vi "HMI_Prototype.vi"() -> ()   [LabVIEW 2014]
uses:
  machineState.ctl
  controls.ctl
  <vilib>/DAQmx/write.llb/DAQmx Write (Digital Bool 1Line 1Point).vi
  <vilib>/DAQmx/read.llb/DAQmx Read (Analog DBL 1Chan 1Samp).vi
  <vilib>/DAQmx/miscellaneous.llb/DAQmx Fill In Error Info.vi
panel:
  out "lab":dbl
  out "solution":dbl
  out "Issue Resolved:":bool
  out "Budget:":dbl=800.0 format="$%#_g.00"
  out "Time Remaining:":timestamp=timestamp(1800 s since 1904-01-01) format="%<%M:%S>T"
  in  "Terminal:":T1(ring)
  in  "Component:":T2(ring)
  in  "Tighten Terminal":bool
  in  "Replace Component":bool
  in  "Segment:":T3(ring)
  in  "Aquire Voltage":bool
  out "Voltage:":dbl
  out "Lab:":string
  in  "Close Lab":bool
  in  "Reset Lab":bool
  out "V+ Solenoid":bool
  out "B+ Solenoid":bool
  out "A- Solenoid":bool
  out "A+ Solenoid":bool
  out "Manual":bool
  out "Auto":bool=TRUE
  out "Stop Button":bool
  out "Start Button":bool
  in  "Tab Control":T4(tab)
  in  "WebBrowser":refnum<k7>(container)
  out "s1":picture
  out "s2":picture
  out "s3":picture
  out "s4":picture
  in  "V+":bool
  in  "B+":bool
  in  "A-":bool
  in  "A+":bool
  in  "START":bool
  in  "AUTO/MAN":bool
  in  "STOP":bool
  # "A+"
  # "A-"
  # "B+"
  # "V+"
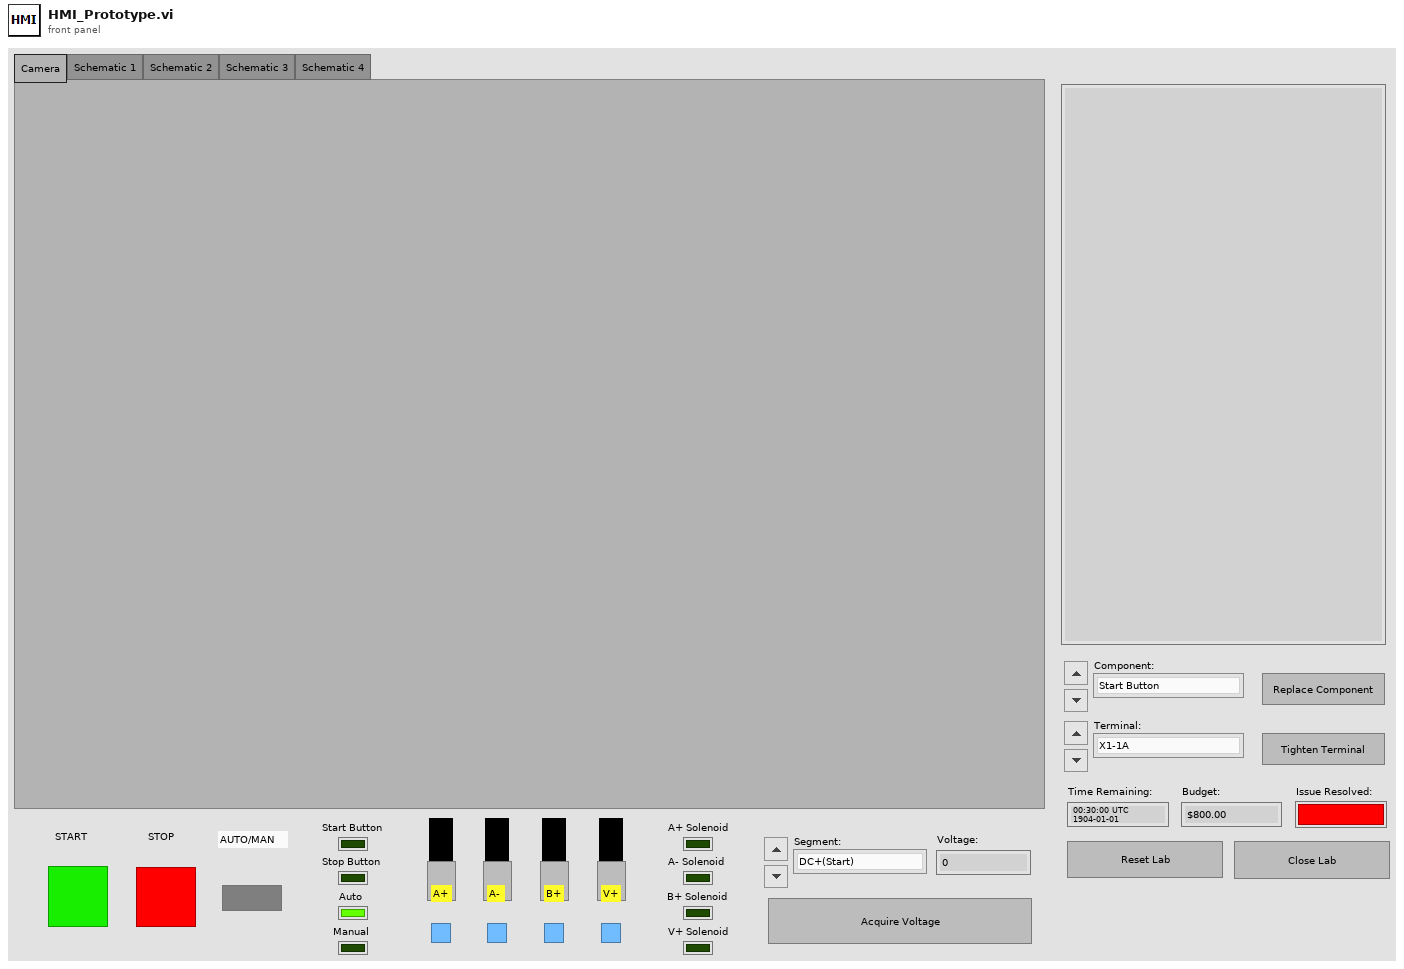
[diagram p1: front panel]
types:
  T1 = enum16{"X1-1A", "X1-2A", "X1-3A", "X1-4A", "X1-5A", "X1-6A", "X1-7A", "X1-8A", "X1-9A", "X1-10A", "X1-11A", "X1-12A", "X1-1B", "X1-2B", "X1-3B", "X1-4B", "X1-5B", "X1-6B", "X1-7B", "X1-8B", "X1-9B", "X1-10B", "X1-11B", "X1-12B", "X1-1C", "X1-2C", "X1-3C", "X1-4C", "X1-5C", "X1-6C", "X1-7C", "X1-8C", "X1-9C", "X1-10C", "X1-11C", "X1-12C", "X1-1D", "X1-2D", "X1-3D", "X1-4D", "X1-5D", "X1-6D", "X1-7D", "X1-8D", "X1-9D", "X1-10D", "X1-11D", "X1-12D", "PLC-VDC(O/0)", "PLC-O/0", "PLC-VDC(O/1)", "PLC-O/1", "PLC-VDC(O/2)", "PLC-O/2", "PLC-VDC(O/3)", "PLC-O/3", "PLC-DC_COM1", "PLC-I/0", "PLC-I/1", "PLC-I/2", "PLC-I/3", "PLC-DC_COM2", "PLC-I/4", "PLC-I/5", "PLC-I/6", "PLC-I/7", "Start Button Terminals", "Stop Button Terminals", "Auto/Man Terminals", "DM1(a0) Terminals", "DM2(a1) Terminals", "DM3(b0) Terminals", "DM4(b1) Terminals", "DM5(v) Terminals", "EL1(A+) Terminals", "EL2(A-) Terminals", "EL3(B+) Terminals", "EL4(V+) Terminals"}
  T2 = enum16{"Start Button", "Stop Button", "Auto/Man Switch", "DM1(a0)", "DM2(a1)", "DM3(b0)", "DM4(b1)", "DM5(v)", "EL1(A+)", "EL2(A-)", "EL3(B+)", "EL4(V+)", "PLC"}
  T3 = enum16{"DC+(Start)", "PB(Start)", "I/0(Start)", "DC+(Stop)", "PB(Stop)", "I/1(Stop)", "DC+(Auto/Man)", "I/2(Auto/Man)", "DC+(a0)", "I/3(a0)", "DC+(a1)", "I/4(a1)", "DC+(b0)", "I/5(b0)", "DC+(b1)", "I/6(b1)", "DC+(v)", "I/7(v)", "DC+(O/0)(VAC/VDC)", "O/0(EL1A+)", "EL1A+(A1)", "EL1A+(A2)", "DC+(O/1)(VAC/VDC)", "O/1(EL2A-)", "EL2A-(A1)", "EL2A-(A2)", "O/2(EL3B+)(A1)", "EL3B+(A2)", "O/3(EL4V+)(A1)", "EL4V+(A2)", "DC-(DC_COM)", "DC-(0V)"}
  T4 = enum32{"Camera", "Schematic 1", "Schematic 2", "Schematic 3", "Schematic 4"}
  T5 = typedef "controls.ctl" = enum16{"Initialize", "Start Button", "Stop Button", "AutoMan Switch", "A Plus Button", "A Minus Button", "B Plus Button", "V Plus Button", "Change View", "Acquire Voltage", "Replace Component", "Tighten Terminal", "Reset Lab", "Close Lab"}
  T6 = typedef "machineState.ctl" = enum16{"idle", "running"}
  T7 = typedef "imagedata.ctl" = cluster{"image type":i32, "image depth":i32, "image":u8[], "mask":u8[], "colors":u32[], "Rectangle":cluster{"left":i16, "top":i16, "right":i16, "bottom":i16}}
  T8 = enum16{"open", "replace", "create", "open or create", "replace or create", "replace or create with confirmation"}
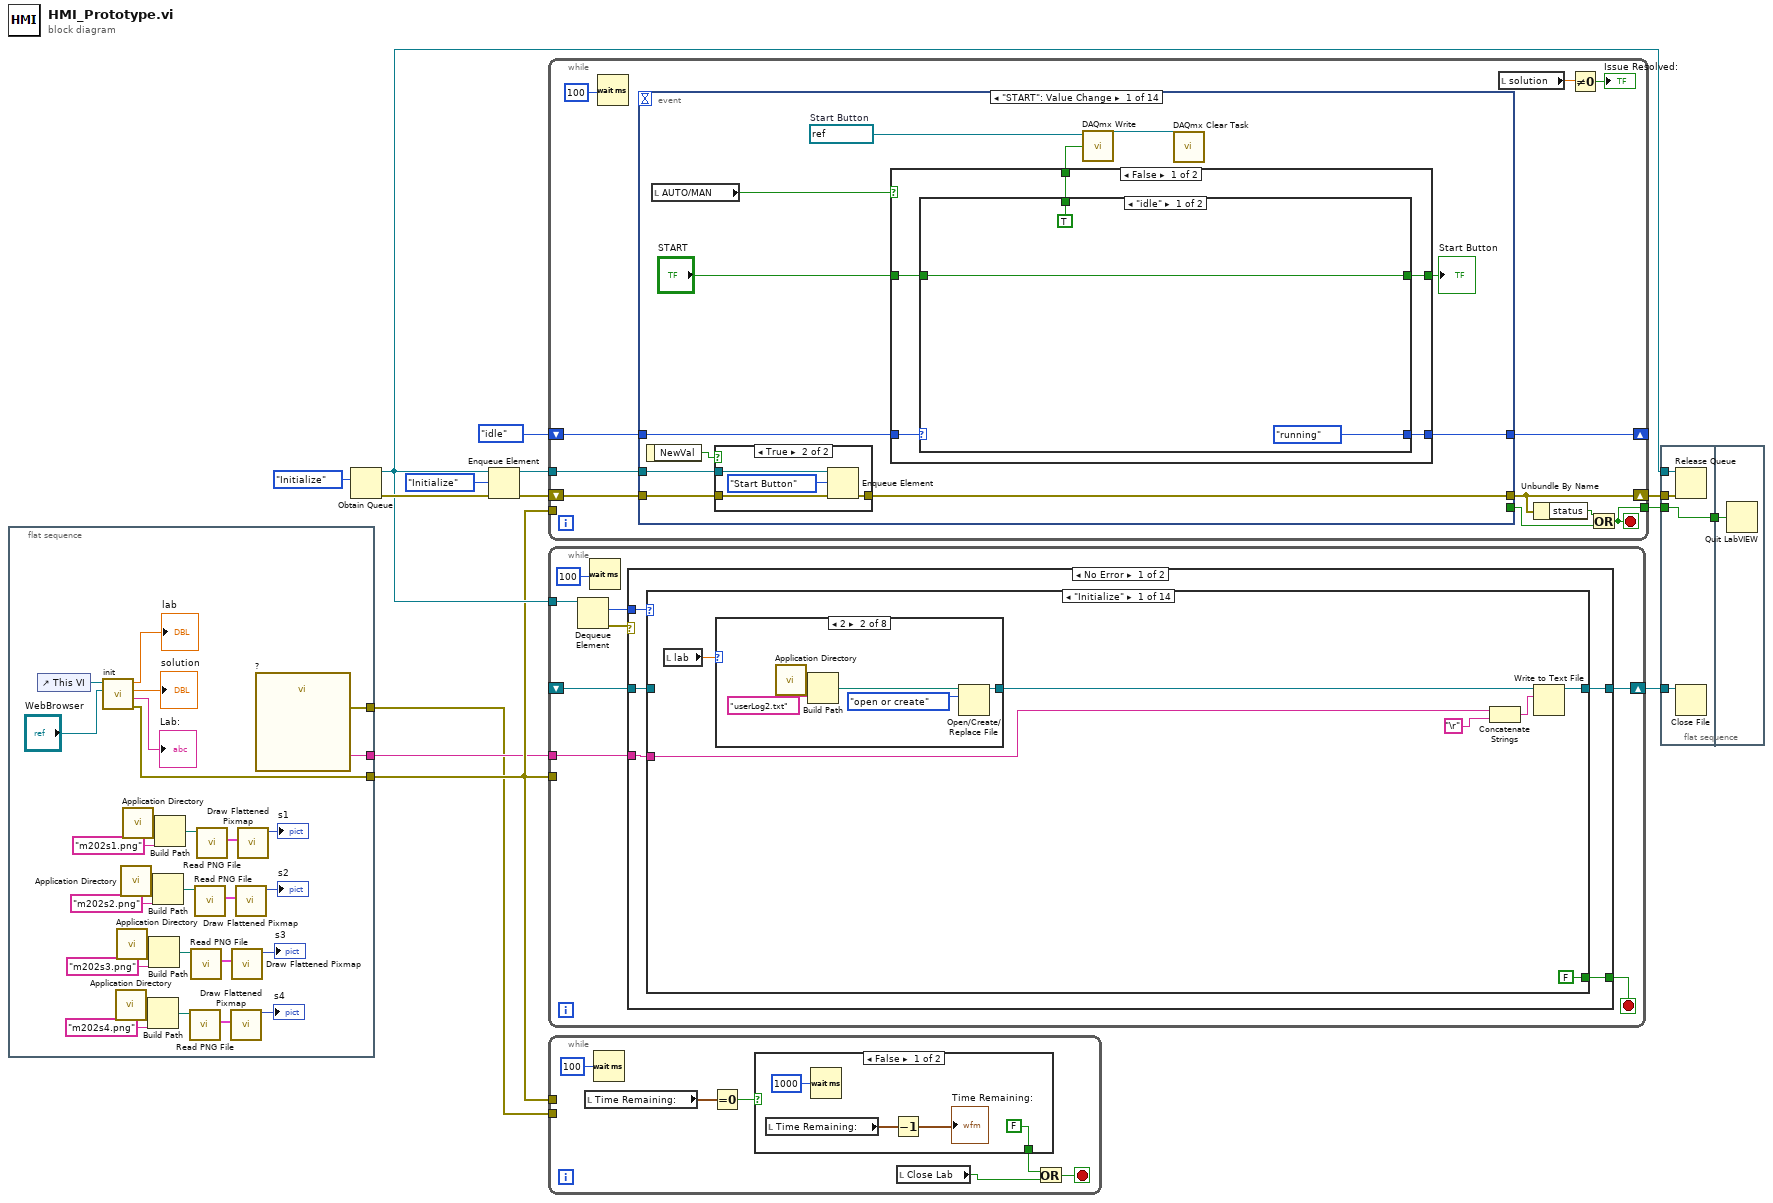
[diagram p0: block diagram]
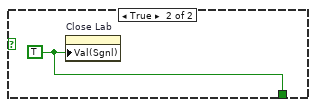
[diagram p2: hidden frame]
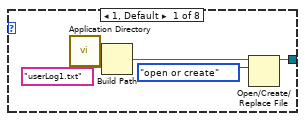
[diagram p3: hidden frame]
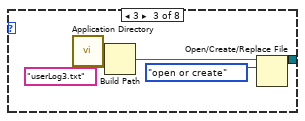
[diagram p4: hidden frame]
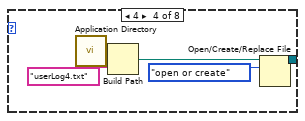
[diagram p5: hidden frame]
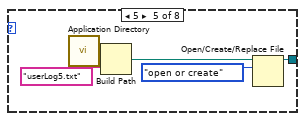
[diagram p6: hidden frame]
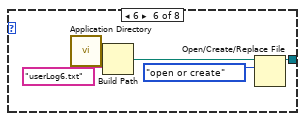
[diagram p7: hidden frame]
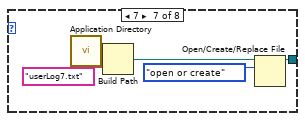
[diagram p8: hidden frame]
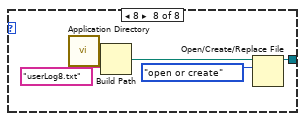
[diagram p9: hidden frame]
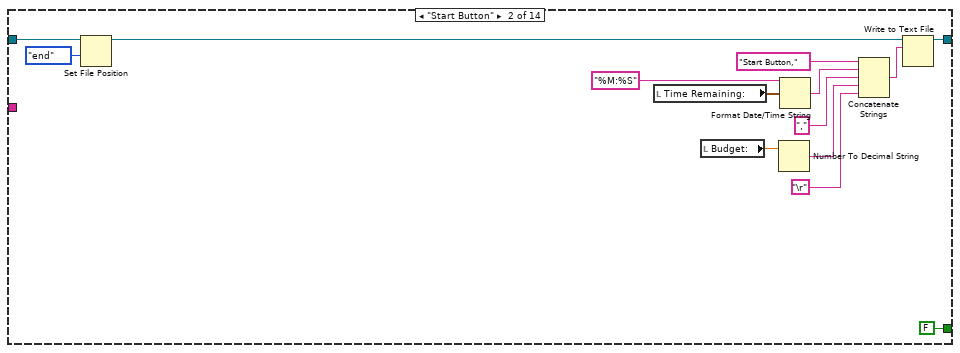
[diagram p10: hidden frame]
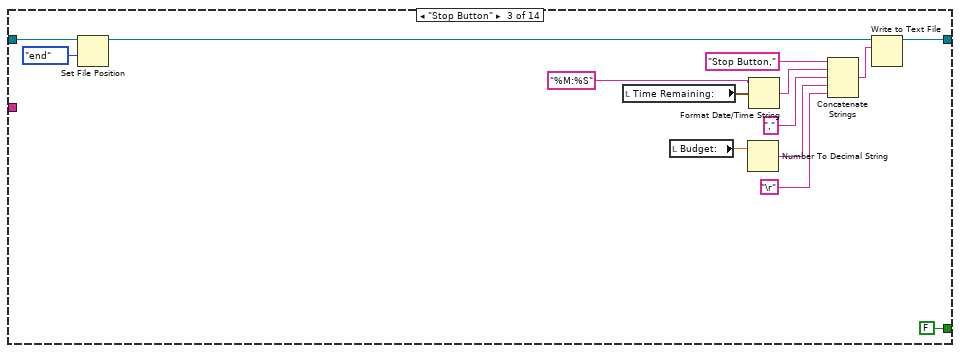
[diagram p11: hidden frame]
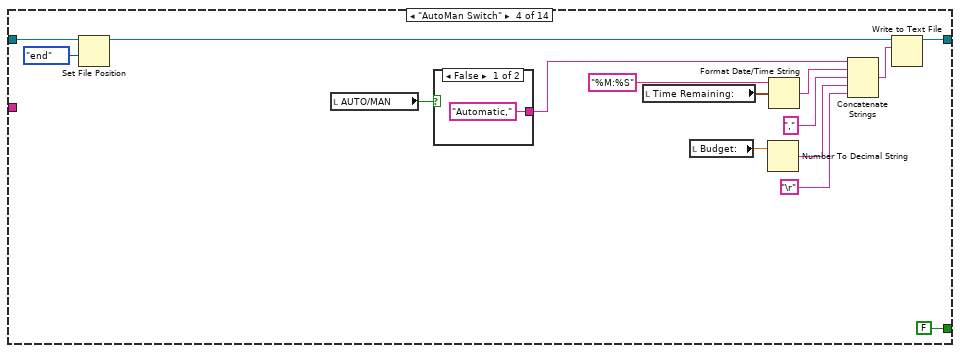
[diagram p12: hidden frame]
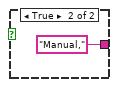
[diagram p13: hidden frame]
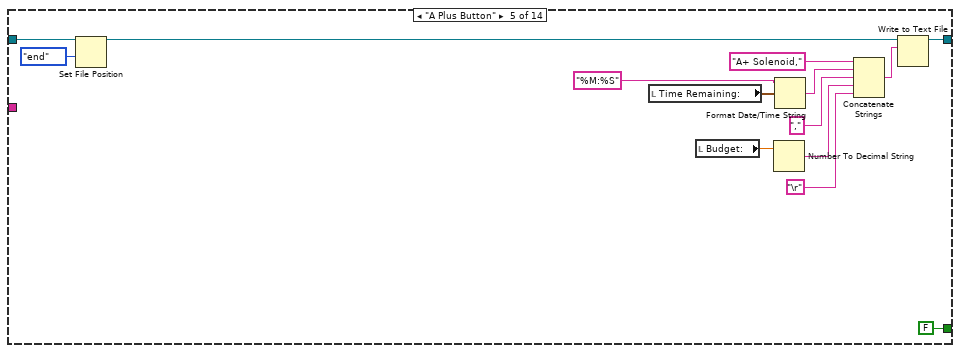
[diagram p14: hidden frame]
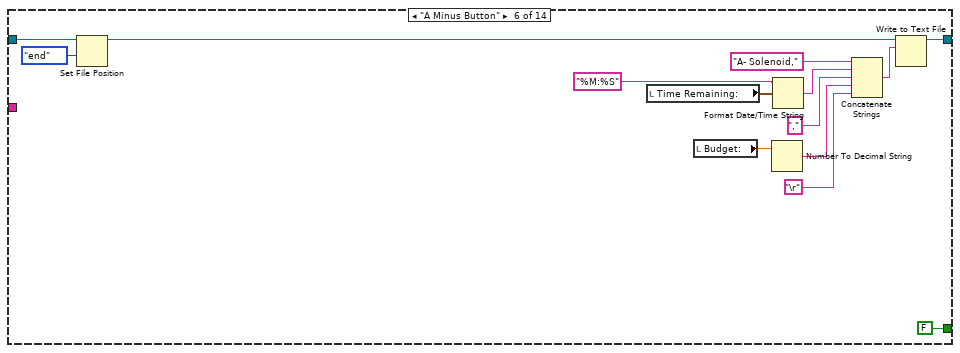
[diagram p15: hidden frame]
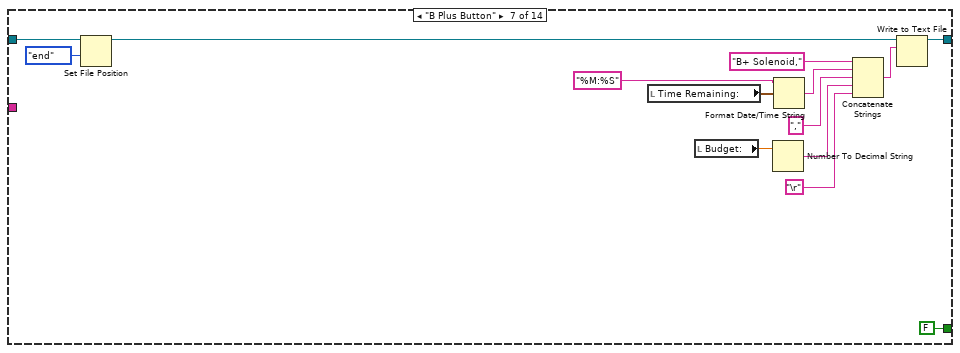
[diagram p16: hidden frame]
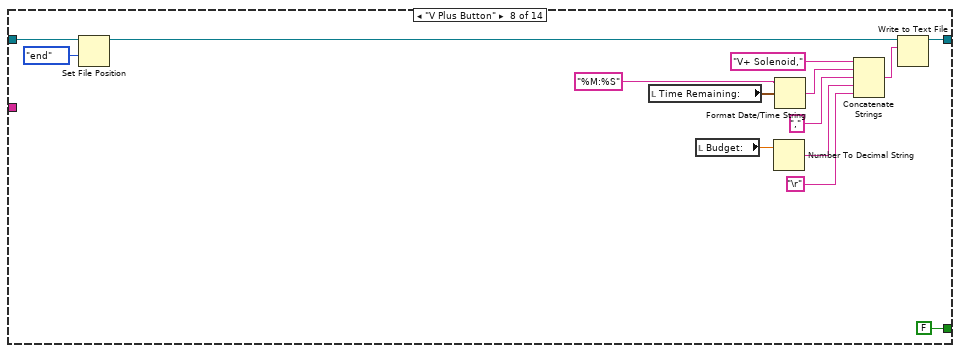
[diagram p17: hidden frame]
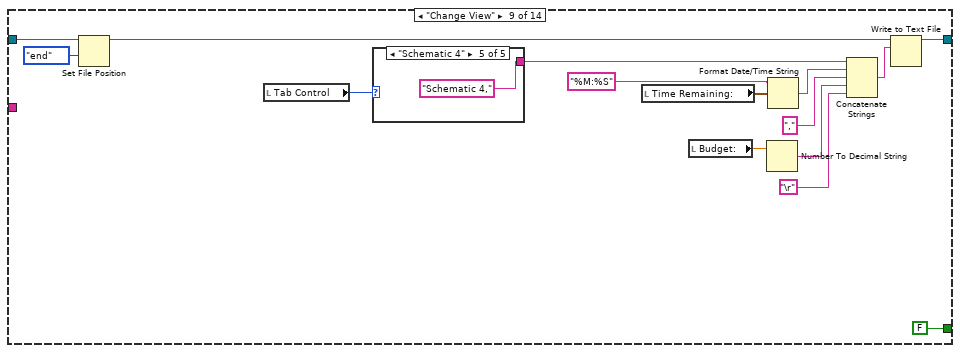
[diagram p18: hidden frame]
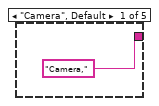
[diagram p19: hidden frame]
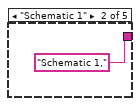
[diagram p20: hidden frame]
diagram:
  n1 = flat-sequence {
    tunnel: [w37] -> w6
    tunnel: [w36] -> w2
    tunnel: [w35] -> w1
    frame #0 {
      n2 = control-ref of="This VI"() -> (w42:refnum<vi>)
      n3 = call "init.vi"("WebBrowser"="WebBrowser", "VI in"=w42) -> ("error out"=w37:errorcluster, "Lab Description:"=→"Lab:":string, "solution"=→"solution":dbl, "lab"=→"lab":dbl)  [unwired: 6 in]
      n4 = call <vilib>:"Application Directory.vi"() -> ("Application Directory"=w21:path)
      n5 = call <vilib>:"Application Directory.vi"() -> ("Application Directory"=w22:path)
      n6 = call <vilib>:"Application Directory.vi"() -> ("Application Directory"=w29:path)
      n7 = call <vilib>:"Application Directory.vi"() -> ("Application Directory"=w30:path)
      n8 = Build Path(base path=w21, name or relative path="m202s4.png") -> (appended path=w18:path)
      n9 = Build Path(base path=w22, name or relative path="m202s3.png") -> (appended path=w25:path)
      n10 = Build Path(base path=w29, name or relative path="m202s2.png") -> (appended path=w26:path)
      n11 = Build Path(base path=w30, name or relative path="m202s1.png") -> (appended path=w33:path)
      n12 = call <vilib>:"Read PNG File.vi"("path to PNG file"=w18) -> ("image data"=w19:T7)  [unwired: 8 in, 2 out]
      n13 = call <vilib>:"Read PNG File.vi"("path to PNG file"=w25) -> ("image data"=w24:T7)  [unwired: 8 in, 2 out]
      n14 = call <vilib>:"Read PNG File.vi"("path to PNG file"=w26) -> ("image data"=w27:T7)  [unwired: 8 in, 2 out]
      n15 = call <vilib>:"Read PNG File.vi"("path to PNG file"=w33) -> ("image data"=w32:T7)  [unwired: 8 in, 2 out]
      n16 = call <vilib>:"Draw Flattened Pixmap.vi"("image data"=w19) -> ("new picture"=→"s4":picture)  [unwired: 8 in]
      n17 = call <vilib>:"Draw Flattened Pixmap.vi"("image data"=w24) -> ("new picture"=→"s3":picture)  [unwired: 8 in]
      n18 = call <vilib>:"Draw Flattened Pixmap.vi"("image data"=w27) -> ("new picture"=→"s2":picture)  [unwired: 8 in]
      n19 = call <vilib>:"Draw Flattened Pixmap.vi"("image data"=w32) -> ("new picture"=→"s1":picture)  [unwired: 8 in]
      n20 = call "?"() -> ("Name:"=w36:string, "error out"=w35:errorcluster)  [unwired: 17 in, 1 out]
    }
  }
  n21 = Obtain Queue(element data type=controls."Initialize") -> (queue out=w7:refnum<queue>, error out=w8:errorcluster)  [unwired: 4 in, 1 out]
  n22 = Enqueue Element(queue=w7, element=controls."Initialize", error in (no error)=w8) -> (queue out=w11:refnum<queue>, error out=w10:errorcluster)  [unwired: 1 in, 1 out]
  n23 = while {
    shift-right: [w48] -> w13
    shift-left: w10 -> [w52]
    tunnel: w11 -> [w51]
    shift-right: [w49] -> _
    shift-left: machineState."idle" -> [w50]
    tunnel: w6 -> [_]
    tunnel: [w43] -> w4
    stop <- w43 stop-if-true
    n24 = Wait (ms)(milliseconds to wait=u32 100 ("millisecond timer value")) -> ()  [unwired: 1 out]
    n25 = event shown="[0] \"START\": Value Change" {
      selector: _ -> [_ _ _ _ _ _ _ _ _ _ _ _ _ _]
      dyn-events: _ -> [_ _ _ _ _ _ _ _ _ _ _ _ _ _]
      timeout: _ -> [_ _ _ _ _ _ _ _ _ _ _ _ _ _]
      tunnel: w52 -> [w65 w92 w101 w114 w129 w145 w159 w175 w180 w227 w233 w443 w554 w585]
      tunnel: [w64 w91 w102 w113 w128 w144 w158 w174 w179 w227 w232 w442 w553 w583] -> w48
      tunnel: w51 -> [w63 w90 w100 w115 w130 w143 w160 w176 w181 _ w234 w444 w555 w584]
      tunnel: w50 -> [w57 w87 w104 w112 w127 w142 w157 w172 w178 w228 w231 w441 w552 w581]
      tunnel: [w58 w86 w104 w112 w127 w142 w157 w172 w178 w228 w231 w441 w552 w581] -> w49
      tunnel: [_ _ _ _ _ _ _ _ _ _ _ _ _ w579] -> w46
      event "START": Value Change {
        w60 = refnum<k21> "DO1P0"  # Start Button
        n26 = event-data() -> ("NewVal"=w54:bool)  [unwired: 1 in]
        n27 = local read "AUTO/MAN"() -> (w62:bool)
        n28 = case shown="True" w54 {
          tunnel: w65 -> [w66 w70]
          tunnel: [w66 w69] -> w64
          tunnel: w63 -> [_ w68]
          frame False {
          }
          frame True {
            n29 = Enqueue Element(queue=w68, element=controls."Start Button", error in (no error)=w70) -> (error out=w69:errorcluster)  [unwired: 1 in, 2 out]
          }
        }
        n30 = case shown="False" w62 {
          tunnel: [w73 w83] -> w59
          tunnel: [w74 w82] -> w58
          tunnel: w57 -> [w75 w82]
          tunnel: "START" -> [w71 w83]
          tunnel: [w72 w83] -> w55
          frame False {
            n31 = case shown="\"idle\"" w75 {
              selector: w75 -> [_ w81]
              tunnel: [machineState."running" w81] -> w74
              tunnel: [TRUE ("START") FALSE ("START")] -> w73
              tunnel: [w76 w79] -> w72
              tunnel: w71 -> [w76 w79]
              frame "idle" {
              }
              frame "running" {
              }
            }
          }
          frame True {
          }
        }
        "Start Button" <- w55
        n32 = call-poly <vilib>:"DAQmx Write.vi"("task/channels in"=w60, "data"=w59) -> ("task out"=w61:refnum<k21>)  [unwired: 11 in, 2 out]
        n33 = call <vilib>:"DAQmx Clear Task.vi"("task in"=w61) -> ()  [unwired: 14 in, 1 out]
      }
      event "STOP": Value Change {
        w88 = refnum<k21> "DO1P1"  # Stop Button
        n34 = event-data() -> ("NewVal"=w85:bool)  [unwired: 1 in]
        n35 = case shown="True" w85 {
          tunnel: w92 -> [w93 w97]
          tunnel: [w93 w96] -> w91
          tunnel: w90 -> [_ w95]
          frame False {
          }
          frame True {
            n36 = Enqueue Element(queue=w95, element=controls."Stop Button", error in (no error)=w97) -> (error out=w96:errorcluster)  [unwired: 1 in, 2 out]
          }
        }
        n37 = case shown="\"running\"" w87 {
          selector: w87 -> [w98 _]
          tunnel: [w98 machineState."idle"] -> w86
          frame "idle" {
          }
          frame "running" {
          }
        }
        n38 = call-poly <vilib>:"DAQmx Write.vi"("task/channels in"=w88, "data"="STOP") -> ("task out"=w89:refnum<k21>)  [unwired: 11 in, 2 out]
        n39 = call <vilib>:"DAQmx Clear Task.vi"("task in"=w89) -> ()  [unwired: 14 in, 1 out]
        "Stop Button" <- "STOP"
      }
      event "AUTO/MAN": Value Change {
        n40 = event-data() -> ()  [unwired: 1 in, 1 out]
        n41 = case shown="\"idle\"" w104 {
          frame "idle" {
            w106 = refnum<k21> "DO1P2"  # Auto/Man
            n42 = Equal?(x="AUTO/MAN", y=FALSE) -> (x = y?=→"Auto":bool)
            n43 = call-poly <vilib>:"DAQmx Write.vi"("task/channels in"=w106, "data"="AUTO/MAN") -> ("task out"=w107:refnum<k21>)  [unwired: 11 in, 2 out]
            n44 = call <vilib>:"DAQmx Clear Task.vi"("task in"=w107) -> ()  [unwired: 14 in, 1 out]
            "Manual" <- "AUTO/MAN"
          }
          frame "running" {
            n45 = One Button Dialog(message="The machine is still running.  Please\nstop the machine before switching\nit into 'Manual' mode." ("button name (\"OK\")")) -> ()  [unwired: 1 in, 1 out]
            n46 = invoke on="AUTO/MAN" class="Bool (strict)" method="Reinit To Default"() -> ()  [unwired: 3 in, 3 out]
          }
        }
        n47 = Enqueue Element(queue=w100, element=controls."AutoMan Switch", error in (no error)=w101) -> (error out=w102:errorcluster)  [unwired: 1 in, 2 out]
      }
      event "A+": Value Change {
        n48 = event-data() -> ("NewVal"=w111:bool)  [unwired: 1 in]
        n49 = case shown="True" w111 {
          tunnel: w115 -> [_ w120]
          tunnel: w114 -> [w116 w119]
          tunnel: [w116 w118] -> w113
          frame False {
          }
          frame True {
            n50 = Enqueue Element(queue=w120, element=controls."A Plus Button", error in (no error)=w119) -> (error out=w118:errorcluster)  [unwired: 1 in, 2 out]
          }
        }
        n51 = case shown="\"idle\"" w112 {
          frame "idle" {
            w122 = refnum<k21> "DO1P3"  # A+ Solenoid
            n52 = call-poly <vilib>:"DAQmx Write.vi"("task/channels in"=w122, "data"="A+") -> ("task out"=w123:refnum<k21>)  [unwired: 11 in, 2 out]
            n53 = call <vilib>:"DAQmx Clear Task.vi"("task in"=w123) -> ()  [unwired: 14 in, 1 out]
            "A+ Solenoid" <- "A+"
          }
          frame "running" {
            n54 = local read "A+"() -> (w124:bool)
            n55 = case shown="True" w124 {
              frame False {
              }
              frame True {
                n56 = One Button Dialog(message="The machine is still running. Please\nstop the machine before using\nthe solenoid controls.") -> ()  [unwired: 1 in, 1 out]
              }
            }
          }
        }
      }
      event "A-": Value Change {
        n57 = event-data() -> ("NewVal"=w126:bool)  [unwired: 1 in]
        n58 = case shown="True" w126 {
          tunnel: w130 -> [_ w135]
          tunnel: w129 -> [w131 w134]
          tunnel: [w131 w133] -> w128
          frame False {
          }
          frame True {
            n59 = Enqueue Element(queue=w135, element=controls."A Minus Button", error in (no error)=w134) -> (error out=w133:errorcluster)  [unwired: 1 in, 2 out]
          }
        }
        n60 = case shown="\"idle\"" w127 {
          frame "idle" {
            w137 = refnum<k21> "DO1P4"  # A- Solenoid
            n61 = call-poly <vilib>:"DAQmx Write.vi"("task/channels in"=w137, "data"="A-") -> ("task out"=w138:refnum<k21>)  [unwired: 11 in, 2 out]
            n62 = call <vilib>:"DAQmx Clear Task.vi"("task in"=w138) -> ()  [unwired: 14 in, 1 out]
            "A- Solenoid" <- "A-"
          }
          frame "running" {
            n63 = local read "A-"() -> (w139:bool)
            n64 = case shown="True" w139 {
              frame False {
              }
              frame True {
                n65 = One Button Dialog(message="The machine is still running. Please\nstop the machine before using\nthe solenoid controls.") -> ()  [unwired: 1 in, 1 out]
              }
            }
          }
        }
      }
      event "B+": Value Change {
        n66 = event-data() -> ("NewVal"=w141:bool)  [unwired: 1 in]
        n67 = case shown="True" w141 {
          tunnel: w145 -> [w146 w150]
          tunnel: [w146 w149] -> w144
          tunnel: w143 -> [_ w148]
          frame False {
          }
          frame True {
            n68 = Enqueue Element(queue=w148, element=controls."B Plus Button", error in (no error)=w150) -> (error out=w149:errorcluster)  [unwired: 1 in, 2 out]
          }
        }
        n69 = case shown="\"running\"" w142 {
          frame "idle" {
            w152 = refnum<k21> "DO1P5"  # B+ Solenoid
            n70 = call-poly <vilib>:"DAQmx Write.vi"("task/channels in"=w152, "data"="B+") -> ("task out"=w153:refnum<k21>)  [unwired: 11 in, 2 out]
            n71 = call <vilib>:"DAQmx Clear Task.vi"("task in"=w153) -> ()  [unwired: 14 in, 1 out]
            "B+ Solenoid" <- "B+"
          }
          frame "running" {
            n72 = local read "B+"() -> (w154:bool)
            n73 = case shown="True" w154 {
              frame False {
              }
              frame True {
                n74 = One Button Dialog(message="The machine is still running. Please\nstop the machine before using\nthe solenoid controls.") -> ()  [unwired: 1 in, 1 out]
              }
            }
          }
        }
      }
      event "V+": Value Change {
        n75 = event-data() -> ("NewVal"=w156:bool)  [unwired: 1 in]
        n76 = case shown="True" w156 {
          tunnel: w160 -> [_ w165]
          tunnel: w159 -> [w161 w164]
          tunnel: [w161 w163] -> w158
          frame False {
          }
          frame True {
            n77 = Enqueue Element(queue=w165, element=controls."V Plus Button", error in (no error)=w164) -> (error out=w163:errorcluster)  [unwired: 1 in, 2 out]
          }
        }
        n78 = case shown="\"running\"" w157 {
          frame "idle" {
            w167 = refnum<k21> "DO1P6"  # V+ Solenoid
            n79 = call-poly <vilib>:"DAQmx Write.vi"("task/channels in"=w167, "data"="V+") -> ("task out"=w168:refnum<k21>)  [unwired: 11 in, 2 out]
            n80 = call <vilib>:"DAQmx Clear Task.vi"("task in"=w168) -> ()  [unwired: 14 in, 1 out]
            "V+ Solenoid" <- "V+"
          }
          frame "running" {
            n81 = local read "V+"() -> (w169:bool)
            n82 = case shown="False" w169 {
              frame False {
              }
              frame True {
                n83 = One Button Dialog(message="The machine is still running. Please\nstop the machine before using\nthe solenoid controls.") -> ()  [unwired: 1 in, 1 out]
              }
            }
          }
        }
      }
      event "Tab Control": Value Change {
        n84 = event-data() -> ()  [unwired: 1 in, 1 out]
        n85 = case shown="\"Schematic 1\"" "Tab Control" {
          frame "Camera", Default {
          }
          frame "Schematic 1" {
          }
          frame "Schematic 2" {
          }
          frame "Schematic 3" {
          }
          frame "Schematic 4" {
          }
        }
        n86 = Enqueue Element(queue=w176, element=controls."Change View", error in (no error)=w175) -> (error out=w174:errorcluster)  [unwired: 1 in, 2 out]
      }
      event "Aquire Voltage": Value Change {
        n87 = event-data() -> ("NewVal"=w177:bool)  [unwired: 1 in]
        n88 = while {
          stop <- w187 stop-if-true
          n89 = case shown="True" "Aquire Voltage" {
            tunnel: [TRUE FALSE] -> w187
            frame False {
            }
            frame True {
              n90 = case shown="\"DC-(DC_COM)\"" "Segment:" {
                tunnel: [w195 w196 w197 w198 w199 w200 w201 w202 w203 w204 w205 w206 w207 w208 w209 w210 w211 w212 w213 w214 w215 w216 w217 w218 w219 w220 w221 w222 w223 w224 w225 w226] -> w192
                frame "DC+(Start)" {
                  w195 = refnum<k21> "ACH00"  # DC+(Start)
                }
                frame "PB(Start)" {
                  w196 = refnum<k21> "ACH01"  # PB(Start)
                }
                frame "I/0(Start)" {
                  w197 = refnum<k21> "ACH02"  # I/0(Start)
                }
                frame "DC+(Stop)" {
                  w198 = refnum<k21> "ACH03"  # DC+(Stop)
                }
                frame "PB(Stop)" {
                  w199 = refnum<k21> "ACH04"  # PB(Stop)
                }
                frame "I/1(Stop)" {
                  w200 = refnum<k21> "ACH05"  # I/1(Stop)
                }
                frame "DC+(Auto/Man)" {
                  w201 = refnum<k21> "ACH06"  # DC+(Auto/Man)
                }
                frame "I/2(Auto/Man)" {
                  w202 = refnum<k21> "ACH07"  # I/2(Auto/Man)
                }
                frame "DC+(a0)" {
                  w203 = refnum<k21> "ACH08"  # DC+(A0)
                }
                frame "I/3(a0)" {
                  w204 = refnum<k21> "ACH09"  # I/3(A0)
                }
                frame "DC+(a1)" {
                  w205 = refnum<k21> "ACH10"  # DC+(A1)
                }
                frame "I/4(a1)" {
                  w206 = refnum<k21> "ACH11"  # I/4(A1)
                }
                frame "DC+(b0)" {
                  w207 = refnum<k21> "ACH12"  # DC+(B0)
                }
                frame "I/5(b0)" {
                  w208 = refnum<k21> "ACH13"  # I/5(B0)
                }
                frame "DC+(b1)" {
                  w209 = refnum<k21> "ACH14"  # DC+(B1)
                }
                frame "I/6(b1)" {
                  w210 = refnum<k21> "ACH15"  # I/6(B1)
                }
                frame "DC+(v)" {
                  w211 = refnum<k21> "ACH16"  # DC+(V)
                }
                frame "I/7(v)" {
                  w212 = refnum<k21> "ACH17"  # I/7(V)
                }
                frame "DC+(O/0)(VAC/VDC)" {
                  w213 = refnum<k21> "ACH18"  # DC+(O/0)(VAC/VDC)
                }
                frame "O/0(EL1A+)" {
                  w214 = refnum<k21> "ACH19"  # O/0(EL1A+)
                }
                frame "EL1A+(A1)" {
                  w215 = refnum<k21> "ACH20"  # EL1A+(A1)
                }
                frame "EL1A+(A2)" {
                  w216 = refnum<k21> "ACH21"  # EL1A+(A2)
                }
                frame "DC+(O/1)(VAC/VDC)" {
                  w217 = refnum<k21> "ACH22"  # DC+(O/1)(VAC/VDC)
                }
                frame "O/1(EL2A-)" {
                  w218 = refnum<k21> "ACH23"  # O/1(EL2A-)
                }
                frame "EL2A-(A1)" {
                  w219 = refnum<k21> "ACH24"  # EL2A-(A1)
                }
                frame "EL2A-(A2)" {
                  w220 = refnum<k21> "ACH25"  # EL2A-(A2)
                }
                frame "O/2(EL3B+)(A1)" {
                  w221 = refnum<k21> "ACH26"  # O/2(EL3B+)(A1)
                }
                frame "EL3B+(A2)" {
                  w222 = refnum<k21> "ACH27"  # EL3B+(A2)
                }
                frame "O/3(EL4V+)(A1)" {
                  w223 = refnum<k21> "ACH28"  # O/3(EL4V+)(A1)
                }
                frame "EL4V+(A2)" {
                  w224 = refnum<k21> "ACH29"  # EL4V+(A2)
                }
                frame "DC-(DC_COM)" {
                  w225 = refnum<k21> "ACH30"  # DC-(DC_COM)
                }
                frame "DC-(0V)" {
                  w226 = refnum<k21> "ACH31"  # DC-(0V)
                }
              }
              n91 = call-poly <vilib>:"DAQmx Read.vi"("task/channels in"=w192) -> ("task out"=w193:refnum<k21>, "data"=→"Voltage:":dbl)  [unwired: 12 in, 1 out]
              n92 = call <vilib>:"DAQmx Clear Task.vi"("task in"=w193) -> ()  [unwired: 14 in, 1 out]
            }
          }
        }
        n93 = case shown="True" w177 {
          tunnel: w181 -> [_ w186]
          tunnel: w180 -> [w182 w185]
          tunnel: [w182 w184] -> w179
          frame False {
          }
          frame True {
            n94 = Enqueue Element(queue=w186, element=controls."Acquire Voltage", error in (no error)=w185) -> (error out=w184:errorcluster)  [unwired: 1 in, 2 out]
          }
        }
      }
      event "Segment:": Value Change {
        n95 = event-data() -> ()  [unwired: 1 in, 1 out]
        n96 = invoke on="Voltage:" class="DigNum (strict)" method="Reinit To Default"() -> ()  [unwired: 3 in, 3 out]
      }
      event "Replace Component": Value Change {
        n97 = event-data() -> ()  [unwired: 1 in, 1 out]
        n98 = case shown="True" "Replace Component" {
          tunnel: [FALSE ("T button?") w241] -> w229
          frame False {
          }
          frame True {
            n99 = local read "Budget:"() -> (w242:dbl)
            n100 = case shown="\"EL4(V+)\"" "Component:" {
              tunnel: w242 -> [w247 w266 w285 w295 w304 w323 w342 w352 w362 w381 w391 w410 w420]
              tunnel: [w244 w263 w282 w292 w302 w321 w340 w350 w360 w379 w389 w408 w418] -> w241
              frame "Start Button" {
                n101 = Greater Or Equal?(x=w247, y=20.0) -> (x >= y?=w245:bool)
                n102 = case shown="True" w245 {
                  tunnel: [FALSE ("T button?") w250] -> w244
                  frame False {
                    n103 = One Button Dialog(message="You don't have enough money left in the budget.") -> ()  [unwired: 1 in, 1 out]
                  }
                  frame True {
                    n104 = call "replaceStartDialog.vi"() -> ("T button?"=w250:bool)  [unwired: 11 in]
                    n105 = case shown="True" w250 {
                      frame False {
                      }
                      frame True {
                        n106 = local read "Budget:"() -> (w261:dbl)
                        n107 = local read "solution"() -> (w259:dbl)
                        n108 = local read "lab"() -> (w252:dbl)
                        n109 = Subtract(x=w261, y=20.0) -> (x-y=w262:dbl)
                        n110 = Equal To 0?(x=w259) -> (x = 0?=w254:bool)
                        n111 = Equal?(x=w252, y=1.0) -> (x = y?=w253:bool)
                        n112 = local write "Budget:"(w262) -> ()
                        n113 = And(x=w254, y=w253) -> (x .and. y?=w255:bool)
                        n114 = local read "solution"() -> (w256:dbl)
                        n115 = call "turnOffFault1.vi"() -> ()  [unwired: 12 in]
                        n116 = Select(t=1.0, s=w255, f=w256) -> (s? t:f=w257:dbl)
                        n117 = local write "solution"(w257) -> ()
                      }
                    }
                  }
                }
              }
              frame "Stop Button" {
                n118 = Greater Or Equal?(x=w266, y=20.0) -> (x >= y?=w264:bool)
                n119 = case shown="True" w264 {
                  tunnel: [FALSE ("T button?") w269] -> w263
                  frame False {
                    n120 = One Button Dialog(message="You don't have enough money left in the budget.") -> ()  [unwired: 1 in, 1 out]
                  }
                  frame True {
                    n121 = call "replaceStopDialog.vi"() -> ("T button?"=w269:bool)  [unwired: 11 in]
                    n122 = case shown="True" w269 {
                      frame False {
                      }
                      frame True {
                        n123 = local read "Budget:"() -> (w281:dbl)
                        n124 = local read "solution"() -> (w278:dbl)
                        n125 = local read "lab"() -> (w271:dbl)
                        n126 = Subtract(x=w281, y=20.0) -> (x-y=w279:dbl)
                        n127 = Equal To 0?(x=w278) -> (x = 0?=w273:bool)
                        n128 = Equal?(x=w271, y=3.0) -> (x = y?=w272:bool)
                        n129 = local write "Budget:"(w279) -> ()
                        n130 = And(x=w273, y=w272) -> (x .and. y?=w274:bool)
                        n131 = local read "solution"() -> (w275:dbl)
                        n132 = Select(t=1.0, s=w274, f=w275) -> (s? t:f=w276:dbl)
                        n133 = call "turnOffFault3.vi"() -> ()  [unwired: 12 in]
                        n134 = local write "solution"(w276) -> ()
                      }
                    }
                  }
                }
              }
              frame "Auto/Man Switch" {
                n135 = Greater Or Equal?(x=w285, y=30.0) -> (x >= y?=w283:bool)
                n136 = case shown="True" w283 {
                  tunnel: [FALSE ("T button?") w288] -> w282
                  frame False {
                    n137 = One Button Dialog(message="You don't have enough money left in the budget.") -> ()  [unwired: 1 in, 1 out]
                  }
                  frame True {
                    n138 = call "replaceAutoManDialog.vi"() -> ("T button?"=w288:bool)  [unwired: 11 in]
                    n139 = case shown="True" w288 {
                      frame False {
                      }
                      frame True {
                        n140 = local read "Budget:"() -> (w290:dbl)
                        n141 = Subtract(x=w290, y=30.0) -> (x-y=w289:dbl)
                        n142 = local write "Budget:"(w289) -> ()
                      }
                    }
                  }
                }
              }
              frame "DM1(a0)" {
                n143 = Greater Or Equal?(x=w295, y=120.0) -> (x >= y?=w293:bool)
                n144 = case shown="True" w293 {
                  tunnel: [FALSE ("T button?") w298] -> w292
                  frame False {
                    n145 = One Button Dialog(message="You don't have enough money left in the budget.") -> ()  [unwired: 1 in, 1 out]
                  }
                  frame True {
                    n146 = call "replaceDM1Dialog.vi"() -> ("T button?"=w298:bool)  [unwired: 11 in]
                    n147 = case shown="True" w298 {
                      frame False {
                      }
                      frame True {
                        n148 = local read "Budget:"() -> (w300:dbl)
                        n149 = Subtract(x=w300, y=120.0) -> (x-y=w299:dbl)
                        n150 = local write "Budget:"(w299) -> ()
                      }
                    }
                  }
                }
              }
              frame "DM2(a1)" {
                n151 = Greater Or Equal?(x=w304, y=120.0) -> (x >= y?=w303:bool)
                n152 = case shown="True" w303 {
                  tunnel: [FALSE ("T button?") w308] -> w302
                  frame False {
                    n153 = One Button Dialog(message="You don't have enough money left in the budget.") -> ()  [unwired: 1 in, 1 out]
                  }
                  frame True {
                    n154 = call "replaceDM2Dialog.vi"() -> ("T button?"=w308:bool)  [unwired: 11 in]
                    n155 = case shown="True" w308 {
                      frame False {
                      }
                      frame True {
                        n156 = local read "solution"() -> (w309:dbl)
                        n157 = local read "lab"() -> (w316:dbl)
                        n158 = local read "Budget:"() -> (w319:dbl)
                        n159 = Equal To 0?(x=w309) -> (x = 0?=w314:bool)
                        n160 = Equal?(x=w316, y=4.0) -> (x = y?=w315:bool)
                        n161 = Subtract(x=w319, y=120.0) -> (x-y=w318:dbl)
                        n162 = And(x=w314, y=w315) -> (x .and. y?=w313:bool)
                        n163 = local read "solution"() -> (w312:dbl)
                        n164 = local write "Budget:"(w318) -> ()
                        n165 = Select(t=1.0, s=w313, f=w312) -> (s? t:f=w311:dbl)
                        n166 = call "turnOffFault4.vi"() -> ()  [unwired: 12 in]
                        n167 = local write "solution"(w311) -> ()
                      }
                    }
                  }
                }
              }
              frame "DM3(b0)" {
                n168 = Greater Or Equal?(x=w323, y=120.0) -> (x >= y?=w322:bool)
                n169 = case shown="True" w322 {
                  tunnel: [FALSE ("T button?") w327] -> w321
                  frame False {
                    n170 = One Button Dialog(message="You don't have enough money left in the budget.") -> ()  [unwired: 1 in, 1 out]
                  }
                  frame True {
                    n171 = call "replaceDM3Dialog.vi"() -> ("T button?"=w327:bool)  [unwired: 11 in]
                    n172 = case shown="True" w327 {
                      frame False {
                      }
                      frame True {
                        n173 = local read "solution"() -> (w328:dbl)
                        n174 = local read "lab"() -> (w335:dbl)
                        n175 = local read "Budget:"() -> (w338:dbl)
                        n176 = Equal To 0?(x=w328) -> (x = 0?=w333:bool)
                        n177 = Equal?(x=w335, y=2.0) -> (x = y?=w334:bool)
                        n178 = Subtract(x=w338, y=120.0) -> (x-y=w337:dbl)
                        n179 = And(x=w333, y=w334) -> (x .and. y?=w332:bool)
                        n180 = local read "solution"() -> (w331:dbl)
                        n181 = local write "Budget:"(w337) -> ()
                        n182 = Select(t=3.0, s=w332, f=w331) -> (s? t:f=w330:dbl)
                        n183 = call "turnOffFault2.vi"() -> ()  [unwired: 12 in]
                        n184 = local write "solution"(w330) -> ()
                      }
                    }
                  }
                }
              }
              frame "DM4(b1)" {
                n185 = Greater Or Equal?(x=w342, y=120.0) -> (x >= y?=w341:bool)
                n186 = case shown="True" w341 {
                  tunnel: [FALSE ("T button?") w346] -> w340
                  frame False {
                    n187 = One Button Dialog(message="You don't have enough money left in the budget.") -> ()  [unwired: 1 in, 1 out]
                  }
                  frame True {
                    n188 = call "replaceDM4Dialog.vi"() -> ("T button?"=w346:bool)  [unwired: 11 in]
                    n189 = case shown="True" w346 {
                      frame False {
                      }
                      frame True {
                        n190 = local read "Budget:"() -> (w348:dbl)
                        n191 = Subtract(x=w348, y=120.0) -> (x-y=w347:dbl)
                        n192 = local write "Budget:"(w347) -> ()
                      }
                    }
                  }
                }
              }
              frame "DM5(v)" {
                n193 = Greater Or Equal?(x=w352, y=120.0) -> (x >= y?=w351:bool)
                n194 = case shown="True" w351 {
                  tunnel: [FALSE ("T button?") w356] -> w350
                  frame False {
                    n195 = One Button Dialog(message="You don't have enough money left in the budget.") -> ()  [unwired: 1 in, 1 out]
                  }
                  frame True {
                    n196 = call "replaceDM5Dialog.vi"() -> ("T button?"=w356:bool)  [unwired: 11 in]
                    n197 = case shown="True" w356 {
                      frame False {
                      }
                      frame True {
                        n198 = local read "Budget:"() -> (w357:dbl)
                        n199 = Subtract(x=w357, y=120.0) -> (x-y=w359:dbl)
                        n200 = local write "Budget:"(w359) -> ()
                      }
                    }
                  }
                }
              }
              frame "EL1(A+)" {
                n201 = Greater Or Equal?(x=w362, y=80.0) -> (x >= y?=w361:bool)
                n202 = case shown="True" w361 {
                  tunnel: [FALSE ("T button?") w366] -> w360
                  frame False {
                    n203 = One Button Dialog(message="You don't have enough money left in the budget.") -> ()  [unwired: 1 in, 1 out]
                  }
                  frame True {
                    n204 = call "replaceEL1Dialog.vi"() -> ("T button?"=w366:bool)  [unwired: 11 in]
                    n205 = case shown="True" w366 {
                      frame False {
                      }
                      frame True {
                        n206 = local read "solution"() -> (w367:dbl)
                        n207 = local read "lab"() -> (w374:dbl)
                        n208 = local read "Budget:"() -> (w376:dbl)
                        n209 = Equal To 0?(x=w367) -> (x = 0?=w372:bool)
                        n210 = Equal?(x=w374, y=7.0) -> (x = y?=w373:bool)
                        n211 = Subtract(x=w376, y=80.0) -> (x-y=w378:dbl)
                        n212 = And(x=w372, y=w373) -> (x .and. y?=w371:bool)
                        n213 = local read "solution"() -> (w370:dbl)
                        n214 = local write "Budget:"(w378) -> ()
                        n215 = Select(t=1.0, s=w371, f=w370) -> (s? t:f=w369:dbl)
                        n216 = call "turnOffFault7.vi"() -> ()  [unwired: 12 in]
                        n217 = local write "solution"(w369) -> ()
                      }
                    }
                  }
                }
              }
              frame "EL2(A-)" {
                n218 = Greater Or Equal?(x=w381, y=80.0) -> (x >= y?=w380:bool)
                n219 = case shown="True" w380 {
                  tunnel: [FALSE ("T button?") w385] -> w379
                  frame False {
                    n220 = One Button Dialog(message="You don't have enough money left in the budget.") -> ()  [unwired: 1 in, 1 out]
                  }
                  frame True {
                    n221 = call "replaceEL2Dialog.vi"() -> ("T button?"=w385:bool)  [unwired: 11 in]
                    n222 = case shown="True" w385 {
                      frame False {
                      }
                      frame True {
                        n223 = local read "Budget:"() -> (w386:dbl)
                        n224 = Subtract(x=w386, y=80.0) -> (x-y=w388:dbl)
                        n225 = local write "Budget:"(w388) -> ()
                      }
                    }
                  }
                }
              }
              frame "EL3(B+)" {
                n226 = Greater Or Equal?(x=w391, y=80.0) -> (x >= y?=w390:bool)
                n227 = case shown="True" w390 {
                  tunnel: [FALSE ("T button?") w395] -> w389
                  frame False {
                    n228 = One Button Dialog(message="You don't have enough money left in the budget.") -> ()  [unwired: 1 in, 1 out]
                  }
                  frame True {
                    n229 = call "replaceEL3Dialog.vi"() -> ("T button?"=w395:bool)  [unwired: 11 in]
                    n230 = case shown="True" w395 {
                      frame False {
                      }
                      frame True {
                        n231 = local read "solution"() -> (w396:dbl)
                        n232 = local read "lab"() -> (w403:dbl)
                        n233 = local read "Budget:"() -> (w405:dbl)
                        n234 = Equal To 0?(x=w396) -> (x = 0?=w401:bool)
                        n235 = Equal?(x=w403, y=5.0) -> (x = y?=w402:bool)
                        n236 = Subtract(x=w405, y=80.0) -> (x-y=w407:dbl)
                        n237 = And(x=w401, y=w402) -> (x .and. y?=w400:bool)
                        n238 = local read "solution"() -> (w399:dbl)
                        n239 = local write "Budget:"(w407) -> ()
                        n240 = Select(t=3.0, s=w400, f=w399) -> (s? t:f=w398:dbl)
                        n241 = call "turnOffFault5.vi"() -> ()  [unwired: 12 in]
                        n242 = local write "solution"(w398) -> ()
                      }
                    }
                  }
                }
              }
              frame "EL4(V+)" {
                n243 = Greater Or Equal?(x=w410, y=80.0) -> (x >= y?=w409:bool)
                n244 = case shown="True" w409 {
                  tunnel: [FALSE ("T button?") w414] -> w408
                  frame False {
                    n245 = One Button Dialog(message="You don't have enough money left in the budget.") -> ()  [unwired: 1 in, 1 out]
                  }
                  frame True {
                    n246 = call "replaceEL4Dialog.vi"() -> ("T button?"=w414:bool)  [unwired: 11 in]
                    n247 = case shown="True" w414 {
                      frame False {
                      }
                      frame True {
                        n248 = local read "Budget:"() -> (w415:dbl)
                        n249 = Subtract(x=w415, y=80.0) -> (x-y=w417:dbl)
                        n250 = local write "Budget:"(w417) -> ()
                      }
                    }
                  }
                }
              }
              frame "PLC" {
                n251 = Greater Or Equal?(x=w420, y=600.0) -> (x >= y?=w419:bool)
                n252 = case shown="True" w419 {
                  tunnel: [FALSE ("T button?") w424] -> w418
                  frame False {
                    n253 = One Button Dialog(message="You don't have enough money left in the budget.") -> ()  [unwired: 1 in, 1 out]
                  }
                  frame True {
                    n254 = call "replacePLCDialog.vi"() -> ("T button?"=w424:bool)  [unwired: 11 in]
                    n255 = case shown="True" w424 {
                      frame False {
                      }
                      frame True {
                        n256 = local read "Budget:"() -> (w436:dbl)
                        n257 = local read "solution"() -> (w432:dbl)
                        n258 = local read "lab"() -> (w425:dbl)
                        n259 = Subtract(x=w436, y=600.0) -> (x-y=w438:dbl)
                        n260 = Or(x=6.0 ("y"), y=8.0) -> (x .or. y?=w433:i32)
                        n261 = Equal To 0?(x=w432) -> (x = 0?=w427:bool)
                        n262 = Equal?(x=w425, y=w433) -> (x = y?=w426:bool)
                        n263 = local write "Budget:"(w438) -> ()
                        n264 = And(x=w427, y=w426) -> (x .and. y?=w428:bool)
                        n265 = local read "solution"() -> (w429:dbl)
                        n266 = call "turnOffFault6.vi"() -> ()  [unwired: 12 in]
                        n267 = Select(t=1.0, s=w428, f=w429) -> (s? t:f=w430:dbl)
                        n268 = call "turnOffFault8.vi"() -> ()  [unwired: 12 in]
                        n269 = local write "solution"(w430) -> ()
                      }
                    }
                  }
                }
              }
            }
          }
        }
        n270 = case shown="True" w229 {
          tunnel: w234 -> [_ w239]
          tunnel: w233 -> [w235 w238]
          tunnel: [w235 w237] -> w232
          frame False {
          }
          frame True {
            n271 = Enqueue Element(queue=w239, element=controls."Replace Component", error in (no error)=w238) -> (error out=w237:errorcluster)  [unwired: 1 in, 2 out]
          }
        }
      }
      event "Tighten Terminal": Value Change {
        n272 = event-data() -> ("NewVal"=w439:bool)  [unwired: 1 in]
        n273 = case shown="True" w439 {
          tunnel: w444 -> [_ w449]
          tunnel: w443 -> [w445 w448]
          tunnel: [w445 w447] -> w442
          frame False {
          }
          frame True {
            n274 = Enqueue Element(queue=w449, element=controls."Tighten Terminal", error in (no error)=w448) -> (error out=w447:errorcluster)  [unwired: 1 in, 2 out]
          }
        }
        n275 = case shown="True" "Tighten Terminal" {
          frame False {
          }
          frame True {
            n276 = case shown="\"PLC-VDC(O/1)\"" "Terminal:" {
              frame "X1-1A" {
              }
              frame "X1-2A" {
              }
              frame "X1-3A" {
              }
              frame "X1-4A" {
              }
              frame "X1-5A" {
              }
              frame "X1-6A" {
              }
              frame "X1-7A" {
              }
              frame "X1-8A" {
              }
              frame "X1-9A" {
                n277 = call "turnOffFault7.vi"() -> ()  [unwired: 12 in]
                n278 = local read "solution"() -> (w451:dbl)
                n279 = local read "lab"() -> (w458:dbl)
                n280 = Equal To 0?(x=w451) -> (x = 0?=w456:bool)
                n281 = Equal?(x=w458, y=7.0) -> (x = y?=w457:bool)
                n282 = And(x=w456, y=w457) -> (x .and. y?=w455:bool)
                n283 = local read "solution"() -> (w454:dbl)
                n284 = Select(t=2.0, s=w455, f=w454) -> (s? t:f=w453:dbl)
                n285 = local write "solution"(w453) -> ()
              }
              frame "X1-10A" {
              }
              frame "X1-11A" {
              }
              frame "X1-12A" {
              }
              frame "X1-1B" {
                n286 = call "turnOffFault1.vi"() -> ()  [unwired: 12 in]
                n287 = local read "solution"() -> (w460:dbl)
                n288 = local read "lab"() -> (w467:dbl)
                n289 = Equal To 0?(x=w460) -> (x = 0?=w465:bool)
                n290 = Equal?(x=w467, y=1.0) -> (x = y?=w466:bool)
                n291 = And(x=w465, y=w466) -> (x .and. y?=w464:bool)
                n292 = local read "solution"() -> (w463:dbl)
                n293 = Select(t=2.0, s=w464, f=w463) -> (s? t:f=w462:dbl)
                n294 = local write "solution"(w462) -> ()
              }
              frame "X1-2B" {
                n295 = call "turnOffFault3.vi"() -> ()  [unwired: 12 in]
                n296 = local read "solution"() -> (w469:dbl)
                n297 = local read "lab"() -> (w476:dbl)
                n298 = Equal To 0?(x=w469) -> (x = 0?=w474:bool)
                n299 = Equal?(x=w476, y=3.0) -> (x = y?=w475:bool)
                n300 = And(x=w474, y=w475) -> (x .and. y?=w473:bool)
                n301 = local read "solution"() -> (w472:dbl)
                n302 = Select(t=2.0, s=w473, f=w472) -> (s? t:f=w471:dbl)
                n303 = local write "solution"(w471) -> ()
              }
              frame "X1-3B" {
              }
              frame "X1-4B" {
              }
              frame "X1-5B" {
                n304 = call "turnOffFault4.vi"() -> ()  [unwired: 12 in]
                n305 = local read "solution"() -> (w478:dbl)
                n306 = local read "lab"() -> (w485:dbl)
                n307 = Equal To 0?(x=w478) -> (x = 0?=w483:bool)
                n308 = Equal?(x=w485, y=4.0) -> (x = y?=w484:bool)
                n309 = And(x=w483, y=w484) -> (x .and. y?=w482:bool)
                n310 = local read "solution"() -> (w481:dbl)
                n311 = Select(t=2.0, s=w482, f=w481) -> (s? t:f=w480:dbl)
                n312 = local write "solution"(w480) -> ()
              }
              frame "X1-6B" {
              }
              frame "X1-7B" {
              }
              frame "X1-8B" {
              }
              frame "X1-9B" {
              }
              frame "X1-10B" {
              }
              frame "X1-11B" {
              }
              frame "X1-12B" {
              }
              frame "X1-1C" {
              }
              frame "X1-2C" {
              }
              frame "X1-3C" {
              }
              frame "X1-4C" {
              }
              frame "X1-5C" {
              }
              frame "X1-6C" {
              }
              frame "X1-7C" {
              }
              frame "X1-8C" {
              }
              frame "X1-9C" {
              }
              frame "X1-10C" {
                n313 = call "turnOffFault6.vi"() -> ()  [unwired: 12 in]
                n314 = local read "solution"() -> (w487:dbl)
                n315 = local read "lab"() -> (w494:dbl)
                n316 = Equal To 0?(x=w487) -> (x = 0?=w492:bool)
                n317 = Equal?(x=w494, y=6.0) -> (x = y?=w493:bool)
                n318 = And(x=w492, y=w493) -> (x .and. y?=w491:bool)
                n319 = local read "solution"() -> (w490:dbl)
                n320 = Select(t=2.0, s=w491, f=w490) -> (s? t:f=w489:dbl)
                n321 = local write "solution"(w489) -> ()
              }
              frame "X1-11C" {
              }
              frame "X1-12C" {
              }
              frame "X1-1D" {
              }
              frame "X1-2D" {
              }
              frame "X1-3D" {
              }
              frame "X1-4D" {
              }
              frame "X1-5D" {
              }
              frame "X1-6D" {
              }
              frame "X1-7D" {
              }
              frame "X1-8D" {
              }
              frame "X1-9D" {
              }
              frame "X1-10D" {
              }
              frame "X1-11D" {
              }
              frame "X1-12D" {
              }
              frame "PLC-VDC(O/0)" {
              }
              frame "PLC-O/0" {
              }
              frame "PLC-VDC(O/1)" {
                n322 = call "turnOffFault8.vi"() -> ()  [unwired: 12 in]
                n323 = local read "solution"() -> (w496:dbl)
                n324 = local read "lab"() -> (w503:dbl)
                n325 = Equal To 0?(x=w496) -> (x = 0?=w501:bool)
                n326 = Equal?(x=w503, y=8.0) -> (x = y?=w502:bool)
                n327 = And(x=w501, y=w502) -> (x .and. y?=w500:bool)
                n328 = local read "solution"() -> (w499:dbl)
                n329 = Select(t=3.0, s=w500, f=w499) -> (s? t:f=w498:dbl)
                n330 = local write "solution"(w498) -> ()
              }
              frame "PLC-O/1" {
              }
              frame "PLC-VDC(O/2)" {
              }
              frame "PLC-O/2" {
              }
              frame "PLC-VDC(O/3)" {
              }
              frame "PLC-O/3" {
              }
              frame "PLC-DC_COM1" {
                n331 = call "turnOffFault6.vi"() -> ()  [unwired: 12 in]
                n332 = local read "solution"() -> (w505:dbl)
                n333 = local read "lab"() -> (w512:dbl)
                n334 = Equal To 0?(x=w505) -> (x = 0?=w510:bool)
                n335 = Equal?(x=w512, y=6.0) -> (x = y?=w511:bool)
                n336 = And(x=w510, y=w511) -> (x .and. y?=w509:bool)
                n337 = local read "solution"() -> (w508:dbl)
                n338 = Select(t=3.0, s=w509, f=w508) -> (s? t:f=w507:dbl)
                n339 = local write "solution"(w507) -> ()
              }
              frame "PLC-I/0" {
              }
              frame "PLC-I/1" {
              }
              frame "PLC-I/2" {
              }
              frame "PLC-I/3" {
              }
              frame "PLC-DC_COM2" {
              }
              frame "PLC-I/4" {
              }
              frame "PLC-I/5" {
              }
              frame "PLC-I/6" {
              }
              frame "PLC-I/7" {
              }
              frame "Start Button Terminals" {
                n340 = call "turnOffFault1.vi"() -> ()  [unwired: 12 in]
                n341 = local read "solution"() -> (w514:dbl)
                n342 = local read "lab"() -> (w521:dbl)
                n343 = Equal To 0?(x=w514) -> (x = 0?=w519:bool)
                n344 = Equal?(x=w521, y=1.0) -> (x = y?=w520:bool)
                n345 = And(x=w519, y=w520) -> (x .and. y?=w518:bool)
                n346 = local read "solution"() -> (w517:dbl)
                n347 = Select(t=3.0, s=w518, f=w517) -> (s? t:f=w516:dbl)
                n348 = local write "solution"(w516) -> ()
              }
              frame "Stop Button Terminals" {
                n349 = call "turnOffFault3.vi"() -> ()  [unwired: 12 in]
                n350 = local read "solution"() -> (w523:dbl)
                n351 = local read "lab"() -> (w530:dbl)
                n352 = Equal To 0?(x=w523) -> (x = 0?=w528:bool)
                n353 = Equal?(x=w530, y=3.0) -> (x = y?=w529:bool)
                n354 = And(x=w528, y=w529) -> (x .and. y?=w527:bool)
                n355 = local read "solution"() -> (w526:dbl)
                n356 = Select(t=3.0, s=w527, f=w526) -> (s? t:f=w525:dbl)
                n357 = local write "solution"(w525) -> ()
              }
              frame "Auto/Man Terminals" {
              }
              frame "DM1(a0) Terminals" {
              }
              frame "DM2(a1) Terminals" {
                n358 = call "turnOffFault4.vi"() -> ()  [unwired: 12 in]
                n359 = local read "solution"() -> (w532:dbl)
                n360 = local read "lab"() -> (w539:dbl)
                n361 = Equal To 0?(x=w532) -> (x = 0?=w537:bool)
                n362 = Equal?(x=w539, y=4.0) -> (x = y?=w538:bool)
                n363 = And(x=w537, y=w538) -> (x .and. y?=w536:bool)
                n364 = local read "solution"() -> (w535:dbl)
                n365 = Select(t=3.0, s=w536, f=w535) -> (s? t:f=w534:dbl)
                n366 = local write "solution"(w534) -> ()
              }
              frame "DM3(b0) Terminals" {
              }
              frame "DM4(b1) Terminals" {
              }
              frame "DM5(v) Terminals" {
              }
              frame "EL1(A+) Terminals" {
                n367 = call "turnOffFault7.vi"() -> ()  [unwired: 12 in]
                n368 = local read "solution"() -> (w541:dbl)
                n369 = local read "lab"() -> (w548:dbl)
                n370 = Equal To 0?(x=w541) -> (x = 0?=w546:bool)
                n371 = Equal?(x=w548, y=7.0) -> (x = y?=w547:bool)
                n372 = And(x=w546, y=w547) -> (x .and. y?=w545:bool)
                n373 = local read "solution"() -> (w544:dbl)
                n374 = Select(t=3.0, s=w545, f=w544) -> (s? t:f=w543:dbl)
                n375 = local write "solution"(w543) -> ()
              }
              frame "EL2(A-) Terminals" {
              }
              frame "EL3(B+) Terminals" {
              }
              frame "EL4(V+) Terminals" {
              }
            }
          }
        }
      }
      event "Reset Lab": Value Change {
        n376 = event-data() -> ()  [unwired: 1 in, 1 out]
        n377 = case shown="True" "Reset Lab" {
          tunnel: [FALSE ("T button?") w562] -> w550
          frame False {
          }
          frame True {
            n378 = call "resetLabDialog.vi"() -> ("T button?"=w562:bool)  [unwired: 11 in]
            n379 = case shown="True" w562 {
              frame False {
              }
              frame True {
                n380 = flat-sequence {
                  tunnel: [w565] -> w563
                  tunnel: [w567] -> w564
                  tunnel: w563 -> [w567]
                  tunnel: w564 -> [w568]
                  frame #0 {
                    n381 = local read "lab"() -> (w565:dbl)
                    n382 = call "gracefulShutDown.vi"() -> ()  [unwired: 12 in]
                  }
                  frame #1 {
                    n383 = control-ref of="This VI"() -> (w566:refnum<vi>)
                    n384 = invoke class="VI" method="Default Vals.Reinit All"(reference=w566) -> ()  [unwired: 2 in, 3 out]
                  }
                  frame #2 {
                    n385 = local write "lab"(w568) -> ()
                  }
                  frame #3 {
                    n386 = local read "lab"() -> (w570:dbl)
                    n387 = case shown="2" w570 {
                      tunnel: [w571 w572 w573 w574 w575 w576 w577 w578] -> w569
                      frame 1, Default {
                        n388 = call "turnOnFault1.vi"() -> ()  [unwired: 12 in]
                        n389 = call "lab1Text.vi"() -> ("String"=w571:string)  [unwired: 11 in]
                      }
                      frame 2 {
                        n390 = call "turnOnFault2.vi"() -> ()  [unwired: 12 in]
                        n391 = call "lab2Text.vi"() -> ("String"=w572:string)  [unwired: 11 in]
                      }
                      frame 3 {
                        n392 = call "turnOnFault3.vi"() -> ()  [unwired: 12 in]
                        n393 = call "lab3Text.vi"() -> ("String"=w573:string)  [unwired: 11 in]
                      }
                      frame 4 {
                        n394 = call "turnOnFault4.vi"() -> ()  [unwired: 12 in]
                        n395 = call "lab4Text.vi"() -> ("String"=w574:string)  [unwired: 11 in]
                      }
                      frame 5 {
                        n396 = call "turnOnFault5.vi"() -> ()  [unwired: 12 in]
                        n397 = call "lab5Text.vi"() -> ("String"=w575:string)  [unwired: 11 in]
                      }
                      frame 6 {
                        n398 = call "turnOnFault6.vi"() -> ()  [unwired: 12 in]
                        n399 = call "lab6Text.vi"() -> ("String"=w576:string)  [unwired: 11 in]
                      }
                      frame 7 {
                        n400 = call "turnOnFault7.vi"() -> ()  [unwired: 12 in]
                        n401 = call "lab7Text.vi"() -> ("String"=w577:string)  [unwired: 11 in]
                      }
                      frame 8 {
                        n402 = call "turnOnFault8.vi"() -> ()  [unwired: 12 in]
                        n403 = call "lab8Text.vi"() -> ("String"=w578:string)  [unwired: 11 in]
                      }
                    }
                    n404 = local write "Lab:"(w569) -> ()
                  }
                }
              }
            }
          }
        }
        n405 = case shown="True" w550 {
          tunnel: w555 -> [_ w560]
          tunnel: w554 -> [w556 w559]
          tunnel: [w556 w558] -> w553
          frame False {
          }
          frame True {
            n406 = Enqueue Element(queue=w560, element=controls."Reset Lab", error in (no error)=w559) -> (error out=w558:errorcluster)  [unwired: 1 in, 2 out]
          }
        }
      }
      event "Close Lab": Value Change {
        n407 = event-data() -> ()  [unwired: 1 in, 1 out]
        n408 = case shown="True" "Close Lab" {
          tunnel: [FALSE ("true") w587] -> w579
          frame False {
          }
          frame True {
            n409 = local read "Issue Resolved:"() -> (w588:bool)
            n410 = case shown="True" w588 {
              tunnel: [w590 w591] -> w587
              frame False {
                n411 = One Button Dialog(message="You have failed to resolve the issue in this lab.  ") -> (true=w590:bool)  [unwired: 1 in]
              }
              frame True {
                n412 = local read "solution"() -> (w592:dbl)
                n413 = case shown="1, Default" w592 {
                  tunnel: [w593 w595 w597] -> w591
                  frame 1, Default {
                    n414 = One Button Dialog(message="You have succesfully resolved the issue present in this lab.  However, the component that you replaced wasn't broken.  There were alternative solutions to this lab that didn't require the use of your budget.  Please take a screenshot and send it to your instructor.  ") -> (true=w593:bool)  [unwired: 1 in]
                  }
                  frame 2 {
                    n415 = One Button Dialog(message="You have succesfully resolved the issue present in this lab.  However, there was a more accurate alternative solution available.  Please take a screen shot and send it to your instructor.") -> (true=w595:bool)  [unwired: 1 in]
                  }
                  frame 3 {
                    n416 = One Button Dialog(message="You have succesfully resolved the issue present in this lab.  You have found the best possible solution!  Please take a screen shot and send it to your instructor.") -> (true=w597:bool)  [unwired: 1 in]
                  }
                }
              }
            }
          }
        }
        n417 = Enqueue Element(queue=w584, element=controls."Close Lab", error in (no error)=w585) -> (error out=w583:errorcluster)  [unwired: 1 in, 2 out]
      }
    }
    n418 = local read "solution"() -> (w44:dbl)
    n419 = Unbundle By Name(w48) -> ("status"=w47:bool)
    n420 = Not Equal To 0?(x=w44) -> (x != 0?=→"Issue Resolved:":bool)
    n421 = Or(x=w47, y=w46) -> (x .or. y?=w43:bool)
  }
  n422 = while {
    tunnel: w7 -> [w605]
    tunnel: w6 -> [_]
    shift-right: [w602] -> w3
    shift-left: _ -> [w601]
    tunnel: w2 -> [w599]
    stop <- w600 stop-if-true
    n423 = Dequeue Element(queue=w605) -> (element=w604:T5, error out=w603:errorcluster)  [unwired: 2 in, 2 out]
    n424 = Wait (ms)(milliseconds to wait=u32 100 ("millisecond timer value")) -> ()  [unwired: 1 out]
    n425 = case shown="No Error" w603 {
      tunnel: w604 -> [w611 _]
      tunnel: [w610 TRUE] -> w600
      tunnel: [w609 w980] -> w602
      tunnel: w601 -> [w608 w980]
      tunnel: w599 -> [w607 _]
      frame No Error {
        n426 = case shown="\"Initialize\"" w611 {
          tunnel: [FALSE FALSE FALSE FALSE FALSE FALSE FALSE FALSE FALSE FALSE FALSE FALSE FALSE TRUE] -> w610
          tunnel: [w615 w669 w674 w691 w706 w722 w736 w750 w764 w784 w830 w858 w950 w963] -> w609
          tunnel: w608 -> [_ w670 w684 w699 w715 w720 w734 w748 w772 w792 w839 w867 w959 w964]
          tunnel: w607 -> [w613 _ _ _ _ _ _ _ _ _ _ _ _ _]
          frame "Initialize" {
            n427 = local read "lab"() -> (w617:dbl)
            n428 = case shown="2" w617 {
              tunnel: [w623 w624 w629 w634 w639 w644 w649 w654] -> w614
              frame 1, Default {
                n429 = call <vilib>:"Application Directory.vi"() -> ("Application Directory"=w621:path)
                n430 = Build Path(base path=w621, name or relative path="userLog1.txt") -> (appended path=w619:path)
                n431 = Open/Create/Replace File(file path (use dialog)=w619, operation (0:open)=T8."open or create") -> (refnum out=w623:refnum<file>)  [unwired: 4 in, 2 out]
              }
              frame 2 {
                n432 = call <vilib>:"Application Directory.vi"() -> ("Application Directory"=w626:path)
                n433 = Build Path(base path=w626, name or relative path="userLog2.txt") -> (appended path=w628:path)
                n434 = Open/Create/Replace File(file path (use dialog)=w628, operation (0:open)=T8."open or create") -> (refnum out=w624:refnum<file>)  [unwired: 4 in, 2 out]
              }
              frame 3 {
                n435 = call <vilib>:"Application Directory.vi"() -> ("Application Directory"=w631:path)
                n436 = Build Path(base path=w631, name or relative path="userLog3.txt") -> (appended path=w633:path)
                n437 = Open/Create/Replace File(file path (use dialog)=w633, operation (0:open)=T8."open or create") -> (refnum out=w629:refnum<file>)  [unwired: 4 in, 2 out]
              }
              frame 4 {
                n438 = call <vilib>:"Application Directory.vi"() -> ("Application Directory"=w636:path)
                n439 = Build Path(base path=w636, name or relative path="userLog4.txt") -> (appended path=w638:path)
                n440 = Open/Create/Replace File(file path (use dialog)=w638, operation (0:open)=T8."open or create") -> (refnum out=w634:refnum<file>)  [unwired: 4 in, 2 out]
              }
              frame 5 {
                n441 = call <vilib>:"Application Directory.vi"() -> ("Application Directory"=w641:path)
                n442 = Build Path(base path=w641, name or relative path="userLog5.txt") -> (appended path=w643:path)
                n443 = Open/Create/Replace File(file path (use dialog)=w643, operation (0:open)=T8."open or create") -> (refnum out=w639:refnum<file>)  [unwired: 4 in, 2 out]
              }
              frame 6 {
                n444 = call <vilib>:"Application Directory.vi"() -> ("Application Directory"=w646:path)
                n445 = Build Path(base path=w646, name or relative path="userLog6.txt") -> (appended path=w648:path)
                n446 = Open/Create/Replace File(file path (use dialog)=w648, operation (0:open)=T8."open or create") -> (refnum out=w644:refnum<file>)  [unwired: 4 in, 2 out]
              }
              frame 7 {
                n447 = call <vilib>:"Application Directory.vi"() -> ("Application Directory"=w651:path)
                n448 = Build Path(base path=w651, name or relative path="userLog7.txt") -> (appended path=w653:path)
                n449 = Open/Create/Replace File(file path (use dialog)=w653, operation (0:open)=T8."open or create") -> (refnum out=w649:refnum<file>)  [unwired: 4 in, 2 out]
              }
              frame 8 {
                n450 = call <vilib>:"Application Directory.vi"() -> ("Application Directory"=w656:path)
                n451 = Build Path(base path=w656, name or relative path="userLog8.txt") -> (appended path=w658:path)
                n452 = Open/Create/Replace File(file path (use dialog)=w658, operation (0:open)=T8."open or create") -> (refnum out=w654:refnum<file>)  [unwired: 4 in, 2 out]
              }
            }
            n453 = Concatenate Strings(w613, "\r") -> (w616:string)
            n454 = Write to Text File(file (use dialog)=w614, text=w616) -> (refnum out=w615:refnum<file>)  [unwired: 2 in, 2 out]
          }
          frame "Start Button" {
            n455 = Set File Position(refnum=w670, from (0:start)=enum16{"start", "end", "current"}."end") -> (refnum out=w668:refnum<file>)  [unwired: 2 in, 1 out]
            n456 = local read "Time Remaining:"() -> (w665:timestamp)
            n457 = local read "Budget:"() -> (w662:dbl)
            n458 = Number To Decimal String(number=w662) -> (decimal integer string=w661:string)  [unwired: 1 in]
            n459 = Format Date/Time String(time format string (%c)="%M:%S", seconds (now)=w665) -> (date/time string=w664:string)  [unwired: 1 in]
            n460 = Concatenate Strings("Start Button," ("string"), w664, ",", w661, "\r") -> (w667:string)
            n461 = Write to Text File(file (use dialog)=w668, text=w667) -> (refnum out=w669:refnum<file>)  [unwired: 2 in, 2 out]
          }
          frame "Stop Button" {
            n462 = Set File Position(refnum=w684, from (0:start)=enum16{"start", "end", "current"}."end") -> (refnum out=w675:refnum<file>)  [unwired: 2 in, 1 out]
            n463 = local read "Time Remaining:"() -> (w681:timestamp)
            n464 = local read "Budget:"() -> (w678:dbl)
            n465 = Number To Decimal String(number=w678) -> (decimal integer string=w677:string)  [unwired: 1 in]
            n466 = Format Date/Time String(time format string (%c)="%M:%S", seconds (now)=w681) -> (date/time string=w680:string)  [unwired: 1 in]
            n467 = Concatenate Strings("Stop Button," ("string"), w680, ",", w677, "\r") -> (w683:string)
            n468 = Write to Text File(file (use dialog)=w675, text=w683) -> (refnum out=w674:refnum<file>)  [unwired: 2 in, 2 out]
          }
          frame "AutoMan Switch" {
            n469 = Set File Position(refnum=w699, from (0:start)=enum16{"start", "end", "current"}."end") -> (refnum out=w690:refnum<file>)  [unwired: 2 in, 1 out]
            n470 = local read "AUTO/MAN"() -> (w688:bool)
            n471 = case shown="False" w688 {
              tunnel: ["Automatic," ("string") "Manual," ("string")] -> w689
              frame False {
              }
              frame True {
              }
            }
            n472 = local read "Time Remaining:"() -> (w697:timestamp)
            n473 = local read "Budget:"() -> (w694:dbl)
            n474 = Number To Decimal String(number=w694) -> (decimal integer string=w693:string)  [unwired: 1 in]
            n475 = Format Date/Time String(time format string (%c)="%M:%S", seconds (now)=w697) -> (date/time string=w696:string)  [unwired: 1 in]
            n476 = Concatenate Strings(w689, w696, ",", w693, "\r") -> (w698:string)
            n477 = Write to Text File(file (use dialog)=w690, text=w698) -> (refnum out=w691:refnum<file>)  [unwired: 2 in, 2 out]
          }
          frame "A Plus Button" {
            n478 = Set File Position(refnum=w715, from (0:start)=enum16{"start", "end", "current"}."end") -> (refnum out=w705:refnum<file>)  [unwired: 2 in, 1 out]
            n479 = local read "Time Remaining:"() -> (w712:timestamp)
            n480 = local read "Budget:"() -> (w709:dbl)
            n481 = Number To Decimal String(number=w709) -> (decimal integer string=w708:string)  [unwired: 1 in]
            n482 = Format Date/Time String(time format string (%c)="%M:%S", seconds (now)=w712) -> (date/time string=w711:string)  [unwired: 1 in]
            n483 = Concatenate Strings("A+ Solenoid," ("string"), w711, ",", w708, "\r") -> (w714:string)
            n484 = Write to Text File(file (use dialog)=w705, text=w714) -> (refnum out=w706:refnum<file>)  [unwired: 2 in, 2 out]
          }
          frame "A Minus Button" {
            n485 = Set File Position(refnum=w720, from (0:start)=enum16{"start", "end", "current"}."end") -> (refnum out=w719:refnum<file>)  [unwired: 2 in, 1 out]
            n486 = local read "Time Remaining:"() -> (w728:timestamp)
            n487 = local read "Budget:"() -> (w725:dbl)
            n488 = Number To Decimal String(number=w725) -> (decimal integer string=w724:string)  [unwired: 1 in]
            n489 = Format Date/Time String(time format string (%c)="%M:%S", seconds (now)=w728) -> (date/time string=w727:string)  [unwired: 1 in]
            n490 = Concatenate Strings("A- Solenoid," ("string"), w727, ",", w724, "\r") -> (w730:string)
            n491 = Write to Text File(file (use dialog)=w719, text=w730) -> (refnum out=w722:refnum<file>)  [unwired: 2 in, 2 out]
          }
          frame "B Plus Button" {
            n492 = Set File Position(refnum=w734, from (0:start)=enum16{"start", "end", "current"}."end") -> (refnum out=w733:refnum<file>)  [unwired: 2 in, 1 out]
            n493 = local read "Time Remaining:"() -> (w742:timestamp)
            n494 = local read "Budget:"() -> (w739:dbl)
            n495 = Number To Decimal String(number=w739) -> (decimal integer string=w738:string)  [unwired: 1 in]
            n496 = Format Date/Time String(time format string (%c)="%M:%S", seconds (now)=w742) -> (date/time string=w741:string)  [unwired: 1 in]
            n497 = Concatenate Strings("B+ Solenoid," ("string"), w741, ",", w738, "\r") -> (w744:string)
            n498 = Write to Text File(file (use dialog)=w733, text=w744) -> (refnum out=w736:refnum<file>)  [unwired: 2 in, 2 out]
          }
          frame "V Plus Button" {
            n499 = Set File Position(refnum=w748, from (0:start)=enum16{"start", "end", "current"}."end") -> (refnum out=w747:refnum<file>)  [unwired: 2 in, 1 out]
            n500 = local read "Time Remaining:"() -> (w756:timestamp)
            n501 = local read "Budget:"() -> (w753:dbl)
            n502 = Number To Decimal String(number=w753) -> (decimal integer string=w752:string)  [unwired: 1 in]
            n503 = Format Date/Time String(time format string (%c)="%M:%S", seconds (now)=w756) -> (date/time string=w755:string)  [unwired: 1 in]
            n504 = Concatenate Strings("V+ Solenoid," ("string"), w755, ",", w752, "\r") -> (w758:string)
            n505 = Write to Text File(file (use dialog)=w747, text=w758) -> (refnum out=w750:refnum<file>)  [unwired: 2 in, 2 out]
          }
          frame "Change View" {
            n506 = Set File Position(refnum=w772, from (0:start)=enum16{"start", "end", "current"}."end") -> (refnum out=w763:refnum<file>)  [unwired: 2 in, 1 out]
            n507 = local read "Tab Control"() -> (w762:T4)
            n508 = case shown="\"Schematic 4\"" w762 {
              tunnel: ["Camera," "Schematic 1," "Schematic 2," "Schematic 3," "Schematic 4,"] -> w761
              frame "Camera", Default {
              }
              frame "Schematic 1" {
              }
              frame "Schematic 2" {
              }
              frame "Schematic 3" {
              }
              frame "Schematic 4" {
              }
            }
            n509 = local read "Time Remaining:"() -> (w770:timestamp)
            n510 = local read "Budget:"() -> (w767:dbl)
            n511 = Number To Decimal String(number=w767) -> (decimal integer string=w766:string)  [unwired: 1 in]
            n512 = Format Date/Time String(time format string (%c)="%M:%S", seconds (now)=w770) -> (date/time string=w769:string)  [unwired: 1 in]
            n513 = Concatenate Strings(w761, w769, ",", w766, "\r") -> (w771:string)
            n514 = Write to Text File(file (use dialog)=w763, text=w771) -> (refnum out=w764:refnum<file>)  [unwired: 2 in, 2 out]
          }
          frame "Acquire Voltage" {
            n515 = Set File Position(refnum=w792, from (0:start)=enum16{"start", "end", "current"}."end") -> (refnum out=w783:refnum<file>)  [unwired: 2 in, 1 out]
            n516 = local read "Segment:"() -> (w781:T3)
            n517 = case shown="\"DC+(Start)\", Default" w781 {
              tunnel: ["DC+(Start) measured," ("string") "PB(Start) measured," ("string") "I/0(Start) measured," ("string") "DC+(Stop) measured," ("string") "PB(Stop) measured," ("string") "I/1(Stop) measured," ("string") "DC+(Auto/Man) measured," ("string") "I/2(Auto/Man) measured," ("string") "DC+(a0) measured," ("string") "I/3(a0) measured," ("string") "DC+(a1) measured," ("string") "I/4(a1) measured," ("string") "DC+(b0) measured," ("string") "I/5(b0) measured," ("string") "DC+(b1) measured," ("string") "I/6(b1) measured," ("string") "DC+(v) measured," ("string") "I/7(v) measured," ("string") "DC+(O/0)(VAC/VDC) measured," ("string") "O/0(EL1A+) measured," ("string") "EL1A+(A1) measured," ("string") "EL1A+(A2) measured," ("string") "DC+(O/1)(VAC/VDC) measured," ("string") "O/1(EL2A-) measured," ("string") "EL2A-(A1) measured," ("string") "EL2A-(A2) measured," ("string") "O/2(EL3B+)(A1) measured," ("string") "EL3B+(A2) measured," ("string") "O/3(EL4V+)(A1) measured," ("string") "EL4V+(A2) measured," ("string") "DC-(DC_COM) measured," ("string") "DC-(0V) measured," ("string")] -> w782
              frame "DC+(Start)", Default {
              }
              frame "PB(Start)" {
              }
              frame "I/0(Start)" {
              }
              frame "DC+(Stop)" {
              }
              frame "PB(Stop)" {
              }
              frame "I/1(Stop)" {
              }
              frame "DC+(Auto/Man)" {
              }
              frame "I/2(Auto/Man)" {
              }
              frame "DC+(a0)" {
              }
              frame "I/3(a0)" {
              }
              frame "DC+(a1)" {
              }
              frame "I/4(a1)" {
              }
              frame "DC+(b0)" {
              }
              frame "I/5(b0)" {
              }
              frame "DC+(b1)" {
              }
              frame "I/6(b1)" {
              }
              frame "DC+(v)" {
              }
              frame "I/7(v)" {
              }
              frame "DC+(O/0)(VAC/VDC)" {
              }
              frame "O/0(EL1A+)" {
              }
              frame "EL1A+(A1)" {
              }
              frame "EL1A+(A2)" {
              }
              frame "DC+(O/1)(VAC/VDC)" {
              }
              frame "O/1(EL2A-)" {
              }
              frame "EL2A-(A1)" {
              }
              frame "EL2A-(A2)" {
              }
              frame "O/2(EL3B+)(A1)" {
              }
              frame "EL3B+(A2)" {
              }
              frame "O/3(EL4V+)(A1)" {
              }
              frame "EL4V+(A2)" {
              }
              frame "DC-(DC_COM)" {
              }
              frame "DC-(0V)" {
              }
            }
            n518 = local read "Time Remaining:"() -> (w790:timestamp)
            n519 = local read "Budget:"() -> (w787:dbl)
            n520 = Number To Decimal String(number=w787) -> (decimal integer string=w786:string)  [unwired: 1 in]
            n521 = Format Date/Time String(time format string (%c)="%M:%S", seconds (now)=w790) -> (date/time string=w789:string)  [unwired: 1 in]
            n522 = Concatenate Strings(w782, w789, ",", w786, "\r") -> (w791:string)
            n523 = Write to Text File(file (use dialog)=w783, text=w791) -> (refnum out=w784:refnum<file>)  [unwired: 2 in, 2 out]
          }
          frame "Replace Component" {
            n524 = Set File Position(refnum=w839, from (0:start)=enum16{"start", "end", "current"}."end") -> (refnum out=w829:refnum<file>)  [unwired: 2 in, 1 out]
            n525 = local read "Component:"() -> (w828:T2)
            n526 = case shown="\"Auto/Man Switch\"" w828 {
              tunnel: ["Start Button Replaced," ("string") "Stop Button Replaced," ("string") "Auto/Man Switch Replaced," ("string") "DM1(a0) Replaced," ("string") "DM2(a1) Replaced," ("string") "DM3(b0) Replaced," ("string") "DM4(b1) Replaced," ("string") "DM5(v) Replaced," ("string") "EL1(A+) Replaced," ("string") "EL2(A-) Replaced," ("string") "EL3(B+) Replaced," ("string") "EL4(V+) Replaced," ("string") "PLC Replaced," ("string")] -> w837
              frame "Start Button", Default {
              }
              frame "Stop Button" {
              }
              frame "Auto/Man Switch" {
              }
              frame "DM1(a0)" {
              }
              frame "DM2(a1)" {
              }
              frame "DM3(b0)" {
              }
              frame "DM4(b1)" {
              }
              frame "DM5(v)" {
              }
              frame "EL1(A+)" {
              }
              frame "EL2(A-)" {
              }
              frame "EL3(B+)" {
              }
              frame "EL4(V+)" {
              }
              frame "PLC" {
              }
            }
            n527 = local read "Time Remaining:"() -> (w836:timestamp)
            n528 = local read "Budget:"() -> (w833:dbl)
            n529 = Number To Decimal String(number=w833) -> (decimal integer string=w832:string)  [unwired: 1 in]
            n530 = Format Date/Time String(time format string (%c)="%M:%S", seconds (now)=w836) -> (date/time string=w835:string)  [unwired: 1 in]
            n531 = Concatenate Strings(w837, w835, ",", w832, "\r") -> (w838:string)
            n532 = Write to Text File(file (use dialog)=w829, text=w838) -> (refnum out=w830:refnum<file>)  [unwired: 2 in, 2 out]
          }
          frame "Tighten Terminal" {
            n533 = Set File Position(refnum=w867, from (0:start)=enum16{"start", "end", "current"}."end") -> (refnum out=w857:refnum<file>)  [unwired: 2 in, 1 out]
            n534 = local read "Terminal:"() -> (w856:T1)
            n535 = case shown="\"X1-1A\", Default" w856 {
              tunnel: ["X1-1A tightened," ("string") "X1-2A tightened," ("string") "X1-3A tightened," ("string") "X1-4A tightened," ("string") "X1-5A tightened," ("string") "X1-6A tightened," ("string") "X1-7A tightened," ("string") "X1-8A tightened," ("string") "X1-9A tightened," ("string") "X1-10A tightened," ("string") "X1-11A tightened," ("string") "X1-12A tightened," ("string") "X1-1B tightened," ("string") "X1-2B tightened," ("string") "X1-3B tightened," ("string") "X1-4B tightened," ("string") "X1-5B tightened," ("string") "X1-6B tightened," ("string") "X1-7B tightened," ("string") "X1-8B tightened," ("string") "X1-9B tightened," ("string") "X1-10B tightened," ("string") "X1-11B tightened," ("string") "X1-12B tightened," ("string") "X1-1C tightened," ("string") "X1-2C tightened," ("string") "X1-3C tightened," ("string") "X1-4C tightened," ("string") "X1-5C tightened," ("string") "X1-6C tightened," ("string") "X1-7C tightened," ("string") "X1-8C tightened," ("string") "X1-9C tightened," ("string") "X1-10C tightened," ("string") "X1-11C tightened," ("string") "X1-12C tightened," ("string") "X1-1D tightened," ("string") "X1-2D tightened," ("string") "X1-3D tightened," ("string") "X1-4D tightened," ("string") "X1-5D tightened," ("string") "X1-6D tightened," ("string") "X1-7D tightened," ("string") "X1-8D tightened," ("string") "X1-9D tightened," ("string") "X1-10D tightened," ("string") "X1-11D tightened," ("string") "X1-12D tightened," ("string") "PLC-VDC(O/0) tightened," ("string") "PLC-O/0 tightened," ("string") "PLC-VDC(O/1) tightened," ("string") "PLC-O/1 tightened," ("string") "PLC-VDC(O/2) tightened," ("string") "PLC-O/2 tightened," ("string") "PLC-VDC(O/3) tightened," ("string") "PLC-O/3 tightened," ("string") "PLC-DC_COM1 tightened," ("string") "PLC-I/0 tightened," ("string") "PLC-I/1 tightened," ("string") "PLC-I/2 tightened," ("string") "PLC-I/3 tightened," ("string") "PLC-DC_COM2 tightened," ("string") "PLC-I/4 tightened," ("string") "PLC-I/5 tightened," ("string") "PLC-I/6 tightened," ("string") "PLC-I/7 tightened," ("string") "Start Button Terminals tightened," ("string") "Stop Button Terminals tightened," ("string") "Auto/Man Terminals tightened," ("string") "DM1(a0) Terminals tightened," ("string") "DM2(a1) Terminals tightened," ("string") "DM3(b0) Terminals tightened," ("string") "DM4(b1) tightened," ("string") "DM5(v) Terminals tightened," ("string") "EL1(A+) Terminals tightened," ("string") "EL2(A-) Terminals tightened," ("string") "EL3(B+) Terminals tightened," ("string") "EL4(V+) Terminals tightened," ("string")] -> w865
              frame "X1-1A", Default {
              }
              frame "X1-2A" {
              }
              frame "X1-3A" {
              }
              frame "X1-4A" {
              }
              frame "X1-5A" {
              }
              frame "X1-6A" {
              }
              frame "X1-7A" {
              }
              frame "X1-8A" {
              }
              frame "X1-9A" {
              }
              frame "X1-10A" {
              }
              frame "X1-11A" {
              }
              frame "X1-12A" {
              }
              frame "X1-1B" {
              }
              frame "X1-2B" {
              }
              frame "X1-3B" {
              }
              frame "X1-4B" {
              }
              frame "X1-5B" {
              }
              frame "X1-6B" {
              }
              frame "X1-7B" {
              }
              frame "X1-8B" {
              }
              frame "X1-9B" {
              }
              frame "X1-10B" {
              }
              frame "X1-11B" {
              }
              frame "X1-12B" {
              }
              frame "X1-1C" {
              }
              frame "X1-2C" {
              }
              frame "X1-3C" {
              }
              frame "X1-4C" {
              }
              frame "X1-5C" {
              }
              frame "X1-6C" {
              }
              frame "X1-7C" {
              }
              frame "X1-8C" {
              }
              frame "X1-9C" {
              }
              frame "X1-10C" {
              }
              frame "X1-11C" {
              }
              frame "X1-12C" {
              }
              frame "X1-1D" {
              }
              frame "X1-2D" {
              }
              frame "X1-3D" {
              }
              frame "X1-4D" {
              }
              frame "X1-5D" {
              }
              frame "X1-6D" {
              }
              frame "X1-7D" {
              }
              frame "X1-8D" {
              }
              frame "X1-9D" {
              }
              frame "X1-10D" {
              }
              frame "X1-11D" {
              }
              frame "X1-12D" {
              }
              frame "PLC-VDC(O/0)" {
              }
              frame "PLC-O/0" {
              }
              frame "PLC-VDC(O/1)" {
              }
              frame "PLC-O/1" {
              }
              frame "PLC-VDC(O/2)" {
              }
              frame "PLC-O/2" {
              }
              frame "PLC-VDC(O/3)" {
              }
              frame "PLC-O/3" {
              }
              frame "PLC-DC_COM1" {
              }
              frame "PLC-I/0" {
              }
              frame "PLC-I/1" {
              }
              frame "PLC-I/2" {
              }
              frame "PLC-I/3" {
              }
              frame "PLC-DC_COM2" {
              }
              frame "PLC-I/4" {
              }
              frame "PLC-I/5" {
              }
              frame "PLC-I/6" {
              }
              frame "PLC-I/7" {
              }
              frame "Start Button Terminals" {
              }
              frame "Stop Button Terminals" {
              }
              frame "Auto/Man Terminals" {
              }
              frame "DM1(a0) Terminals" {
              }
              frame "DM2(a1) Terminals" {
              }
              frame "DM3(b0) Terminals" {
              }
              frame "DM4(b1) Terminals" {
              }
              frame "DM5(v) Terminals" {
              }
              frame "EL1(A+) Terminals" {
              }
              frame "EL2(A-) Terminals" {
              }
              frame "EL3(B+) Terminals" {
              }
              frame "EL4(V+) Terminals" {
              }
            }
            n536 = local read "Time Remaining:"() -> (w864:timestamp)
            n537 = local read "Budget:"() -> (w861:dbl)
            n538 = Number To Decimal String(number=w861) -> (decimal integer string=w860:string)  [unwired: 1 in]
            n539 = Format Date/Time String(time format string (%c)="%M:%S", seconds (now)=w864) -> (date/time string=w863:string)  [unwired: 1 in]
            n540 = Concatenate Strings(w865, w863, ",", w860, "\r") -> (w866:string)
            n541 = Write to Text File(file (use dialog)=w857, text=w866) -> (refnum out=w858:refnum<file>)  [unwired: 2 in, 2 out]
          }
          frame "Reset Lab" {
            n542 = Set File Position(refnum=w959, from (0:start)=enum16{"start", "end", "current"}."end") -> (refnum out=w949:refnum<file>)  [unwired: 2 in, 1 out]
            n543 = local read "Time Remaining:"() -> (w956:timestamp)
            n544 = local read "Budget:"() -> (w953:dbl)
            n545 = Number To Decimal String(number=w953) -> (decimal integer string=w952:string)  [unwired: 1 in]
            n546 = Format Date/Time String(time format string (%c)="%M:%S", seconds (now)=w956) -> (date/time string=w955:string)  [unwired: 1 in]
            n547 = Concatenate Strings("Reset Lab," ("string"), w955, ",", w952, "\r") -> (w958:string)
            n548 = Write to Text File(file (use dialog)=w949, text=w958) -> (refnum out=w950:refnum<file>)  [unwired: 2 in, 2 out]
          }
          frame "Close Lab" {
            n549 = flat-sequence {
              tunnel: w964 -> [w977]
              tunnel: [w968] -> w962
              tunnel: [w979] -> w963
              tunnel: w962 -> [w979]
              frame #0 {
                n550 = Set File Position(refnum=w977, from (0:start)=enum16{"start", "end", "current"}."end") -> (refnum out=w967:refnum<file>)  [unwired: 2 in, 1 out]
                n551 = local read "Time Remaining:"() -> (w974:timestamp)
                n552 = local read "Budget:"() -> (w971:dbl)
                n553 = Number To Decimal String(number=w971) -> (decimal integer string=w970:string)  [unwired: 1 in]
                n554 = Format Date/Time String(time format string (%c)="%M:%S", seconds (now)=w974) -> (date/time string=w973:string)  [unwired: 1 in]
                n555 = Concatenate Strings("Lab Closed," ("string"), w973, ",", w970, "\r") -> (w976:string)
                n556 = Write to Text File(file (use dialog)=w967, text=w976) -> (refnum out=w968:refnum<file>)  [unwired: 2 in, 2 out]
              }
              frame #1 {
                n557 = call "gracefulShutDown.vi"() -> ()  [unwired: 12 in]
              }
            }
          }
        }
      }
      frame Error {
      }
    }
  }
  n558 = while {
    tunnel: w6 -> [_]
    tunnel: w1 -> [_]
    stop <- w984 stop-if-true
    n559 = local read "Time Remaining:"() -> (w986:timestamp)
    n560 = Wait (ms)(milliseconds to wait=u32 100) -> ()  [unwired: 1 out]
    n561 = Equal To 0?(x=w986) -> (x = 0?=w985:bool)
    n562 = case shown="False" w985 {
      tunnel: [FALSE w992] -> w983
      frame False {
        n563 = local read "Time Remaining:"() -> (w991:timestamp)
        n564 = Wait (ms)(milliseconds to wait=u32 1000) -> ()  [unwired: 1 out]
        n565 = Decrement(x=w991) -> (x-1=→"Time Remaining:":timestamp)
      }
      frame True {
        w992 = TRUE
        n566 = property on="Close Lab" class="Bool (strict)"("Val(Sgnl)"=w992) -> ()  [unwired: 2 in, 2 out]
      }
    }
    n567 = local read "Close Lab"() -> (w982:bool)
    n568 = Or(x=w983, y=w982) -> (x .or. y?=w984:bool)
  }
  n569 = flat-sequence {
    tunnel: w13 -> [w996]
    tunnel: w7 -> [w995]
    tunnel: [w994] -> w5
    tunnel: w4 -> [w994]
    tunnel: w3 -> [w993]
    tunnel: w5 -> [w997]
    frame #0 {
      n570 = Release Queue(queue=w995, error in (no error)=w996) -> ()  [unwired: 1 in, 3 out]
      n571 = Close File(refnum=w993) -> ()  [unwired: 1 in, 2 out]
    }
    frame #1 {
      n572 = Quit LabVIEW(quit? (T)=w997) -> ()
    }
  }
